vi "UHR-Fleezers Control (fpga) - Boltzmann 04-2018.vi"() -> ()   [LabVIEW 2013]
doc: "UHR-Fleezers Instrument Control Code (fpga)"
uses:
  <vilib>/eio/EIONode/EIONode.xnode
  <vilib>/eio/EIOMethodNode/EIOMethodNode.xnode
  <vilib>/rvi/DataTransferAndStorage/Container/XNode/niFpgaContainer.xnode
  <vilib>/Platform/TimedLoop/XDataNode/XDataNode.xnode
  <vilib>/Platform/TimedLoop/XDataNode/nitl_modes.ctl
  <vilib>/Platform/TimedLoop/XDataNode/XDNodeRunTimeDep.lvlib
  <vilib>/Platform/TimedLoop/XDataNode/wakeup.ctl
  <vilib>/Platform/TimedLoop/XDataNode/timing_clust.ctl
  <vilib>/addons/control/pid/fpga.llb/XNode/niFpgaPID.xnode
  <vilib>/rvi/eio/common/nirviEmuTemplateMethod_errors.vi
  <vilib>/rvi/interface/RandomDataEmulation/nirviRandomDataFpgaReadWriteTemplate.vi
panel:
  in  "Tab Control":T1(tab)=enum."Force FB"
  in  "Set 3":bool
  in  "Set 2":bool=TRUE
  in  "Set 1":bool=TRUE
  in  "Trap Pos to FIFO":bool
  in  "N of AI1 Int Acq Sets":i16=2 min=1 max=3 step=1
  out "AI Late Counter":u8
  in  "ai count":u16=400
  in  "+ phase":bool
  in  "Phase count adjustment":i16
  out "Relative phase":i16
  in  "AI to FIFO":bool
  out "BD1 Frequency Out 1":u64
  out "BD1 Frequency Out 2":u64
  out "Trap Pos FIFO Timeout":u16
  out "Trap AI FIFO Timeout":u16
  in  "Trap FIFO Set Timeout":i32
  in  "Tab Control 2":T2(tab)
  in  "Raster to target force":bool
  out "Actual Scan freq":u64
  out "BD1 measured amplitude 2":u16
  out "BD1 measured amplitude 1":u16
  in  "FB Offset":u16
  in  "FB Multi Factor":i16
  in  "Dynamic FB (Ronen)":bool
  in  "Negate Intensity FB":bool
  in  "RD":bool
  in  "FB1 output high":i16=3000
  in  "FB1 output low":i16
  in  "D1":i16
  in  "I1":i16=5
  in  "P1":i16=10
  in  "Swap F1 and F2":bool
  in  "Cont. Scan":bool
  in  "Abort scan":bool
  in  "Cycles per step":u64
  in  "Scan BD":bool
  in  "Number of scans":u16
  in  "Scan steps":u64
  in  "Scan freq.  increment":i64
  out "Scanning":bool
  in  "Start scan":bool
  in  "OSK Bd 1":bool
  in  "Reset Bd 1":bool
  in  "PMODE":bool
  in  "Direct RF Box \nCommunication":bool
  in  "Data BD 2":u8 format="%08b"
  in  "Data BD 1":u8 format="%08b"
  in  "Address":u8 format="%02x"
  in  "Update Data":bool
  in  "FPGA Controls\n RF Box":bool
  in  "Number Interlace Cycles":u8=2 min=1 max=3
  in  "Interlace Off Parameters":u8=1 min=1 max=3
  in  "Interlace ON/OFF":bool
  out "DIO Relative phase":i16
  in  "Phase count adjustment (DIO)":i16
  in  "+ phase (DIO)":bool
  out "DIO Late Counter":u8
  in  "DIO count 1 (ticks)":u16=400
  in  "DIO count 2 (ticks)":u16=400
  in  "DIO count 3 (ticks)":u16=400
  out "AI2 Y Sum Set 2":i16
  out "AI2 Y Sum Set 1":i16
  in  "FB Setpoint Set 1":i16 min=0 step=1
  in  "FB Reset Set 1":bool
  in  "FB On/Off Set 1":bool
  in  "FB Reset Set 2":bool
  in  "FB On/Off Set 2":bool
  in  "FB Setpoint Set 2":i16 min=0 step=1
  out "Scan I":u64
  in  "Amp switch delay":u8=5
  in  "Raster setpoint":fxp<+/-,16,1>
  in  "XY phase ext loop method":bool
  in  "BD 2 Amplitude 1":u16
  in  "BD 1 Amplitude 1":u16
  in  "BD 2 Frequency 1":u64
  in  "BD 1 Frequency 1":u64
  in  "BD 2 Amplitude 2":u16
  in  "BD 1 Amplitude 2":u16
  in  "BD 2 Frequency 2":u64
  in  "BD 1 Frequency 2":u64
  in  "BD 2 Amplitude 3":u16
  in  "BD 1 Amplitude 3":u16
  in  "BD 2 Frequency 3":u64
  in  "BD 1 Frequency 3":u64
  in  "BD 1 Delay (ticks)":u8
  in  "BD 2 Delay (Ticks)":u8 caption="Count(Ticks)"
  in  "Next trap write delay (ticks)":u8 caption="Count(Ticks)"
  in  "Trap 1 osc enable":bool
  in  "Trap 2 osc enable":bool
  in  "B factor":fxp<+/-,32,16>
  in  "FB Min frequency":u64
  in  "FB Max Frequency":u64
  in  "Dynamic Force FB (Ronen)":bool
  in  "FB2 output high":fxp<+/-,16,1>=0.999969482421875
  in  "FB2 output low":fxp<+/-,16,1>=-1.0
  in  "P2":fxp<+/-,16,8> format="%.11g"
  in  "I2":fxp<+/-,16,8>=10.0 format="%.11g"
  in  "D2":fxp<+/-,16,8> format="%.11g"
  in  "Negate Diff?":bool
  in  "Diff FB Measurement?":bool
  in  "FB Trig Integrate":u32=1
  out "TTrig?":bool
  in  "TTrig Negate Pos":bool=TRUE
  out "Trap Pos FB Int Signal":fxp<+/-,24,9> format="%.18g"
  out "Trap Pos FB Int-Norm Signal":fxp<+/-,16,1> format="%.16g"
  in  "FPGA TTrig Thresh":i64
  in  "FPGA Trap Trig":bool
  out "Trap Pos FB Action":i64
  in  "Trap Pos. FB Offset Factor":i64
  in  "Trap Pos. FB Mult Factor":i64=2
  in  "Trap Pos. FB Reset":bool
  in  "Trap Pos FB Monitor T1 or T2":bool
  in  "AI1 X Scale":u16
  in  "Trap Pos FB Int Count":u16=100
  in  "Trap Pos FB Negate Action":bool
  out "AI1 X Set 2":fxp<+/-,16,1>
  out "AI1 X Set 1":fxp<+/-,16,1>
  in  "Trap Pos. FB SP":fxp<+/-,16,1>
  in  "Force feedback":bool
  out "TTrig Sig":i64
  out "TTrig Fin Thresh":i64
  in  "1D or 2D Scan?":bool
  in  "Abort scan (MCL)":bool
  in  "MCL Scan Axis":bool
  in  "Cont. Scan (MCL)":bool
  out "Scan I (MCL)":u64
  in  "Number of scans (MCL)":u16
  out "Scanning MCL":bool
  in  "Scan steps (MCL)":u64
  in  "Cycles per step (MCL)":u64
  in  "Scan freq.  increment (MCL)":i16
  in  "Start scan (MCL)":bool
  in  "AO2":i16
  in  "AO1":i16
  out "MCL Late Counter":u8
  in  "MCL count":u32=800
  out "MCL Relative Phase":i16
  in  "Phase count adjustment (MCL)":i16
  in  "+ phase (MCL)":bool
  out "APD2 int gate":bool
  out "APD3 out state":bool
  in  "APD Gate Operating Mode":u8 max=2 step=1
  in  "Invert APD Gate":bool
  in  "APD Gate OFF Count":u16=100
  in  "APD Gate ON Count":u16=300
  out "APD 1 Gate Late Counter":u8
  out "APD 1 Gate Relative Phase":i16
  in  "Phase count adjustment (APD 1 Gate)":i16
  in  "+ phase (APD 1 Gate)":bool
  out "APD 2 Counts 0":u32
  out "APD 2 Counts 1":u32
  out "APD 1 Counts 0":u32
  out "APD 1 Counts 1":u32
  out "APD1 out state":bool
  in  "APD AO scale factor":i16=1
  in  "APD to FIFO":bool
  in  "APD Acq Rate Count":u32=20000000
  out "APD Acq Late Counter":u8
  out "APD Acq Relative Phase":i16
  in  "Phase Count Adjustment (APD Acq)":i16
  in  "+ phase (APD Acq)":bool
  in  "Phase count adjustment (APD 2 Gate)":i16
  out "APD 2 Gate Late Counter":u8
  out "APD 2 Gate Relative Phase":i16
  in  "+ phase (APD 2 Gate)":bool
  out "APD2 out state":bool
  out "APD 3 Counts 0":u32
  out "APD 3 Counts 1":u32
  out "APD 3 Gate Late Counter":u8
  in  "Phase count adjustment (APD 3 Gate)":i16
  out "APD 3 Gate Relative Phase":i16
  in  "+ phase (APD 3 Gate)":bool
  out "APD1 int gate":bool
  out "APD3 int gate":bool
  in  "D3":i16
  in  "I3":i16=5
  in  "P3":i16=10
  in  "Green Filter Flipper":bool
  in  "Green FB Count":u16=1200
  out "Green Late Counter":u8
  out "Green FB Relative Phase":i16
  in  "Phase count adjustment (Green FB)":i16=10
  in  "+ phase (Green FB)":bool
  out "Green FB Sum":i16
  in  "Green int current ON count adj":u16=150
  in  "Current Out":u16=30000
  in  "Green FB On/Off":bool
  in  "Green FB Setpoint":i16=250 min=0 step=1
  in  "Green FB Reset":bool
  in  "Operating Mode 2":u8=2 max=2 step=1
  in  "Invert GI 2":bool
  in  "Green interlace OFF count 2":u16=900
  in  "Green interlace ON count 2":u16=300
  out "GI Late Counter 2":u8
  out "GI Relative phase 2":i16
  in  "Phase count adjustment (GI) 2":i16=20
  in  "+ phase (GI) 2":bool
  in  "Green interlace OFF count":u16=100
  out "GI Relative phase":i16
  in  "Phase count adjustment (GI)":i16
  in  "+ phase (GI)":bool
  in  "Green interlace ON count":u16=300
  out "GI Late Counter":u8
  in  "Invert GI":bool
  in  "Operating Mode":u8 max=2 step=1
  in  "+ phase (RI)":bool
  out "RI Relative phase":i16
  out "RI Late Counter":u8
  in  "Red interlace ON count":u16=300
  in  "Red interlace OFF count":u16=100
  in  "Invert RI":bool
  in  "Red Laser Operating Mode":u8 max=2 step=1
  in  "Phase count adjustment (RI)":i16
  out "Red FB Intensity":i16
  in  "RI Current Out":u16=30000
  in  "Red FB On/Off":bool
  in  "D4":i16
  in  "I4":i16=5
  in  "P4":i16=10
  in  "Red FB Setpoint":i16=250 min=0 step=1
  in  "Red FB Reset":bool
  in  "RI Operating Mode 2":u8=2 max=2 step=1
  in  "Invert RI 2":bool
  in  "Phase count adjustment (BI AO)":i16=20
  in  "Blue current ON count adj (AO)":u16=150
  in  "BI Current Out":i16=30000
  in  "Blue FB On/Off":bool
  in  "D5":i16
  in  "I5":i16=5
  in  "P5":i16=10
  in  "Blue FB Setpoint":i16=250 min=0 step=1
  in  "Blue FB Reset":bool
  in  "BI Operating Mode (AO)":u8=2 max=2 step=1
  in  "Invert BI (AO)":bool
  in  "Blue OFF count (AO)":u16=900
  in  "Blue ON count (AO)":u16=300
  out "BI Late Counter (AO)":u8
  out "BI Relative phase (AO)":i16
  in  "+ phase (BI AO)":bool
  in  "Phase count adjustment (BI D)":i16
  in  "Blue Laser Operating Mode (D)":u8 max=2 step=1
  in  "Invert BI (D)":bool
  in  "Blue interlace OFF count (D)":u16=100
  in  "Blue interlace ON count (D)":u16=300
  out "Blue Late Counter (D)":u8
  out "BI Relative phase (D)":i16
  in  "+ phase (BI D)":bool
  out "Blue Intensity":i16
  # "Only one of these can be on\nat a time:"
  # "Raster Scan AOD"
  # "1 (X)"
  # "2 (Y)"
  # "IR Intensity Feedback (RF BD 1)"
  # "FB Gains Set 1"
  # "FB output range 1"
  # "False is usual, True is external loop method"
  # "Parameters if using the external RF switching loop"
  # "Parameters if using the usual internal RF switching method"
  # "FB Triggering Excitation Laser"
  # "Trap Pos. FB Gains"
  # "Trap Pos. FB Range"
  # "AO1 (Y)"
  # "2D"
  # "1D"
  # "AO2 (X)"
  # "APD AO for aligning"
  # "Detection Loop"
  # "Green fluorescent laser digital gate interlacing loop"
  # "0 Forced ON\n1 Forced OFF\n2 Interlacing"
  # "Green FB Gains"
  # "Red fluorescent laser digital gate interlacing loop"
  # "Detection Loop"
  # "0 Forced ON\n1 Forced OFF\n2 Interlacing"
  # "Analog/FB Control Loop\n(Disabled)"
  # "Digital Control Loop"
  # "Blue laser intensity reading"
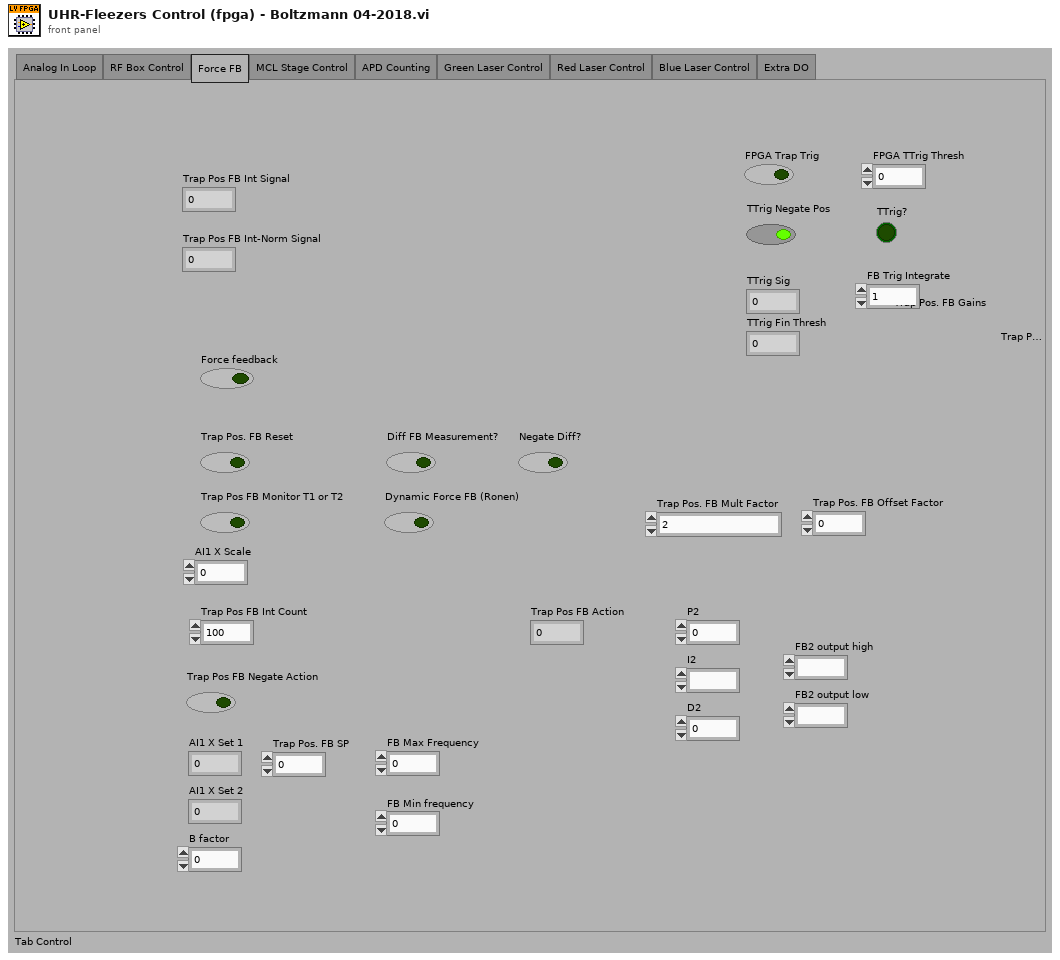
[diagram p1: front panel]
types:
  T1 = enum32{"Analog In Loop", "RF Box Control", "Force FB", "MCL Stage Control", "APD Counting", "Green Laser Control", "Red Laser Control", "Blue Laser Control", "Extra DO"}
  T2 = enum32{"Controls", "Interlacing Frequency and Amplitude Values", "Oscillate trap from memory"}
  T3 = typedef "XDNodeRunTimeDep.lvlib/timing_clust.ctl" = cluster{"Expected End [f-1]":u64, "Actual End [f-1]":u64, "Finished Late? [f-1]":bool, "Expected End [i-1]":u64, "Actual End [i-1]":u64, "Finished Late? [i-1]":bool, "Expected Start [i]":u64, "Actual Start [i]":u64, "Expected Start [f]":u64, "Actual Start [f]":u64, "Source Name":string, "Structure Name":string, "Period":i64, "Deadline":i64, "Offset":i64, "Start":i64, "Priority":i32, "Timeout":i32, "Mode":T4, "Wakeup Reason":T5, "Error":errorcluster, "Source Type":string, "Secondary Source Type":string, "Global End Time":u64, "Global Start Time":u64, "Frame Duration":u64, "Iteration Duration":u64, "Assigned CPU":i32, "I/O Scan Engine Mode":u32}
  T4 = typedef "XDNodeRunTimeDep.lvlib/nitl_modes.ctl" = enum32{"No Change", "Process missed periods, maintain original phase", "Discard missed periods, maintain original phase", "Process missed periods, ignore original phase", "Discard missed periods, ignore original phase"}
  T5 = typedef "XDNodeRunTimeDep.lvlib/wakeup.ctl" = enum32{"Normal", "Aborted", "Asynchronous wakeup", "Timing source error", "Timed loop error", "Timeout"}
  T6 = cluster{"proportional gain (Kc)":i16, "integral gain (Kc*Ts/Ti)":i16, "derivative gain (Kc*Td/Ts)":i16}
  T7 = cluster{"FB1 output high":i16, "FB1 output low":i16}
  T8 = cluster{"P2":fxp<+/-,16,8>, "I2":fxp<+/-,16,8>, "D2":fxp<+/-,16,8>}
  T9 = cluster{"FB2 output high":fxp<+/-,16,1>, "FB2 output low":fxp<+/-,16,1>}
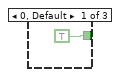
[diagram p2: hidden frame]
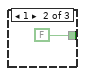
[diagram p3: hidden frame]
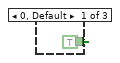
[diagram p4: hidden frame]
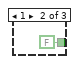
[diagram p5: hidden frame]
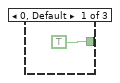
[diagram p7: hidden frame]
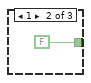
[diagram p8: hidden frame]
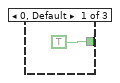
[diagram p10: hidden frame]
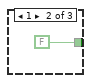
[diagram p11: hidden frame]
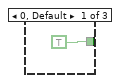
[diagram p14: hidden frame]
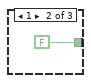
[diagram p15: hidden frame]
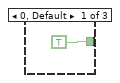
[diagram p17: hidden frame]
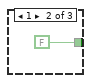
[diagram p18: hidden frame]
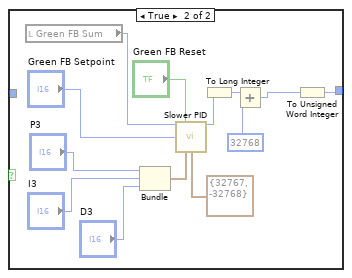
[diagram p20: hidden frame]
diagram:
  w7 = FALSE
  w5 = FALSE
  # "timing array current index"
  # "timing array"
  # "timing counter (phase adjusted here)"
  # "late counter"
  n1 = flat-sequence "FPGA initialization to do before running any of the loops" {
    tunnel: [u16 0 ("DIO count 3 (ticks)")] -> w4
    tunnel: [w15] -> _
    frame #0 {
      w14 = FALSE ("Enable")
      # "BD 2 (Y)"
      # "BD 1 (X)"
      # "Start up expansion chassis early\nto avoid delays later"
      # "This pin controls udclk on the RF boards.\nWhen initially configuring the boards, this pin needs to be\nconfigured as a high impedance input.  Later it will be switched\nto an output."
      # "Initial setting of DIO data and \naddress to low (before reset).  \nThis needs to happen before the other\ncontrol method loops execute."
      n2 = xnode "FPGA I/O Node"("Chassis2/Mod1/AO0"=u16 0 ("Chassis2/Mod4/AO0")) -> ("Chassis2/Mod2/AI0"=w15:i16)  [unwired: 2 in, 2 out]
      n3 = xnode "FPGA I/O Method Node"("Enable"=w14) -> ()  [unwired: 1 in, 1 out]
      n4 = xnode "FPGA I/O Method Node"("Enable"=w14) -> ()  [unwired: 1 in, 1 out]
      n5 = xnode "FPGA I/O Node"("Connector1/DIO0"=FALSE, "Connector1/DIO1"=FALSE, "Connector1/DIO2"=FALSE, "Connector1/DIO3"=FALSE, "Connector1/DIO4"=FALSE, "Connector1/DIO5"=FALSE, "Connector1/DIO6"=FALSE, "Connector1/DIO7"=FALSE, "Connector1/DIO8"=FALSE, "Connector1/DIO9"=FALSE, "Connector1/DIO10"=FALSE, "Connector1/DIO11"=FALSE, "Connector1/DIO12"=FALSE, "Connector1/DIO13"=FALSE, "Connector1/DIO15"=FALSE, "Connector1/DIO20"=FALSE, "Connector1/DIO21"=FALSE, "Connector1/DIO22"=FALSE, "Connector1/DIO23"=FALSE, "Connector1/DIO24"=FALSE, "Connector1/DIO25"=FALSE, "Connector1/DIO26"=FALSE, "Connector1/DIO27"=FALSE, "Connector1/DIO14"=FALSE) -> ()  [unwired: 24 in, 24 out]
    }
  }
  n6 = local read "AO1"() -> (w12:i16)
  n7 = local read "AO2"() -> (w11:i16)
  n8 = node-c288() -> (w10:T3)  [unwired: 1 in]
  n9 = To Unsigned Long Integer(number=w4) -> (unsigned 32bit integer=w8:u32)
  n10 = timed-loop "RF box board DIO control: control bits" {
    timing: w10 -> [_]
    timing-out: [_] -> w9
    tunnel: [w44] -> _
    tunnel: w4 -> [w44]
    stop <- FALSE stop-if-true
    n11 = xnode "FPGA I/O Node"("Connector1/DIO16"="RD", "Connector1/DIO17"="PMODE", "Connector1/DIO18"="OSK Bd 1", "Connector1/DIO19"="Reset Bd 1", "Connector0/DIO3"="Green Filter Flipper") -> ()  [unwired: 5 in, 5 out]
  }
  n12 = disable-structure shown="Disabled" {
    disable-tunnel: w7 -> [w52 _]
    disable-tunnel: w4 -> [w51 _]
    frame Disabled {
      n13 = while "APD 2 Gating" {
        shift-right: [w56] -> _
        shift-left: w51 -> [w61]
        shift-right: [w55] -> _
        shift-left: w52 -> [w53]
        stop <- FALSE stop-if-true
        n14 = flat-sequence {
          tunnel: w61 -> [w64]
          tunnel: [w65] -> w59
          tunnel: [w64] -> w57
          tunnel: [w63] -> w54
          tunnel: w53 -> [w63]
          tunnel: [w68] -> w60
          tunnel: w59 -> [w68]
          tunnel: [w67] -> w58
          tunnel: w57 -> [w67]
          tunnel: w54 -> [w66]
          tunnel: [w90] -> w56
          tunnel: w60 -> [w100]
          tunnel: w58 -> [w98]
          tunnel: [w69] -> w55
          frame #0 {
            n15 = call "Loop Timer8"("Count(Ticks)"=w64) -> ("Tick Count(Ticks)"=w65:u16)
          }
          frame #1 {
            # "Signal maybe then sent through \na transistor before APD"
            n16 = xnode "FPGA I/O Node"("Connector0/DIO8"=w66, "Connector0/DIO9"=w66, "Connector0/DIO10"=w66, "Connector0/DIO11"=w66) -> ()  [unwired: 4 in, 4 out]
            "APD2 int gate" <- w66
          }
          frame #2 {
            n17 = local read "APD Gate ON Count"() -> (w83:u16)
            n18 = local read "APD Gate OFF Count"() -> (w82:u16)
            n19 = feedback #1(TRUE) -> (w95:bool)
            n20 = feedback-in #2(w100) -> ()
            n21 = feedback #2(w100) -> (w84:u16)
            n22 = Not(x=w95) -> (.not. x?=w93:bool)
            n23 = feedback-in #1(w93) -> ()
            n24 = Subtract(x=w100, y=w84) -> (x-y=w99:u16)
            n25 = Select(t=w83, s=w93, f=w82) -> (s? t:f=w97:u16)
            n26 = Subtract(x=w99, y=w98) -> (x-y=w75:u16)
            n27 = Subtract(x=w97, y=w75) -> (x-y=w89:u16)
            n28 = Number To Boolean Array(number=w75) -> (Boolean array=w74:bool[])
            n29 = Or Array Elements(Boolean array=w74) -> (logical OR=w73:bool)
            n30 = Boolean To (0,1)(Boolean="+ phase (APD 2 Gate)") -> (0, 1=w87:i16)
            n31 = Multiply(x=w87, y="Phase count adjustment (APD 2 Gate)") -> (x*y=w85:i16)
            n32 = Boolean To (0,1)(Boolean=w73) -> (0, 1=w80:i16)
            n33 = Add(x=w89, y=w85) -> (x+y=w90:u16)
            n34 = To Unsigned Byte Integer(number=w80) -> (unsigned 8bit integer=w77:u8)
            n35 = feedback #3(i16 0) -> (w92:i16)
            n36 = Subtract(x=w92, y=w85) -> (x-y=w91:i16)
            "APD 2 Gate Relative Phase" <- w91
            n37 = feedback-in #3(w91) -> ()
            n38 = feedback #4(u8 0) -> (w78:u8)
            n39 = Add(x=w77, y=w78) -> (x+y=w76:u8)
            "APD 2 Gate Late Counter" <- w76
            n40 = feedback-in #4(w76) -> ()
            n41 = local read "APD Gate Operating Mode"() -> (w81:u8)
            n42 = case shown="2" w81 {
              tunnel: [TRUE FALSE w103] -> w70
              tunnel: w95 -> [_ _ w103]
              frame 0, Default {
              }
              frame 1 {
              }
              frame 2 {
              }
            }
            n43 = local read "Invert APD Gate"() -> (w72:bool)
            n44 = Not(x=w70) -> (.not. x?=w71:bool)
            n45 = Select(t=w71, s=w72, f=w70) -> (s? t:f=w69:bool)
          }
        }
      }
      n46 = while "APD 1 Gating" {
        shift-right: [w107] -> _
        shift-left: w51 -> [w112]
        shift-right: [w106] -> _
        shift-left: w52 -> [w104]
        stop <- FALSE stop-if-true
        n47 = flat-sequence {
          tunnel: w112 -> [w115]
          tunnel: [w116] -> w110
          tunnel: [w115] -> w108
          tunnel: [w114] -> w105
          tunnel: w104 -> [w114]
          tunnel: [w119] -> w111
          tunnel: w110 -> [w119]
          tunnel: [w118] -> w109
          tunnel: w108 -> [w118]
          tunnel: w105 -> [w117]
          tunnel: [w137] -> w107
          tunnel: w111 -> [w151]
          tunnel: w109 -> [w148]
          tunnel: [w120] -> w106
          frame #0 {
            n48 = call "Loop Timer7"("Count(Ticks)"=w115) -> ("Tick Count(Ticks)"=w116:u16)
          }
          frame #1 {
            # "Signal maybe then sent through \na transistor before APD"
            n49 = xnode "FPGA I/O Node"("Connector0/DIO4"=w117, "Connector0/DIO5"=w117, "Connector0/DIO6"=w117, "Connector0/DIO7"=w117) -> ()  [unwired: 4 in, 4 out]
            "APD1 int gate" <- w117
          }
          frame #2 {
            n50 = feedback #5(TRUE) -> (w143:bool)
            n51 = feedback-in #6(w151) -> ()
            n52 = feedback #6(w151) -> (w150:u16)
            n53 = Not(x=w143) -> (.not. x?=w140:bool)
            n54 = feedback-in #5(w140) -> ()
            n55 = Subtract(x=w151, y=w150) -> (x-y=w149:u16)
            n56 = Select(t="APD Gate ON Count", s=w140, f="APD Gate OFF Count") -> (s? t:f=w145:u16)
            n57 = Subtract(x=w149, y=w148) -> (x-y=w125:u16)
            n58 = Subtract(x=w145, y=w125) -> (x-y=w136:u16)
            n59 = Number To Boolean Array(number=w125) -> (Boolean array=w126:bool[])
            n60 = Or Array Elements(Boolean array=w126) -> (logical OR=w124:bool)
            n61 = Boolean To (0,1)(Boolean="+ phase (APD 1 Gate)") -> (0, 1=w134:i16)
            n62 = Boolean To (0,1)(Boolean=w124) -> (0, 1=w131:i16)
            n63 = Multiply(x=w134, y="Phase count adjustment (APD 1 Gate)") -> (x*y=w132:i16)
            n64 = To Unsigned Byte Integer(number=w131) -> (unsigned 8bit integer=w128:u8)
            n65 = Add(x=w136, y=w132) -> (x+y=w137:u16)
            n66 = feedback #7(i16 0) -> (w139:i16)
            n67 = Subtract(x=w139, y=w132) -> (x-y=w138:i16)
            "APD 1 Gate Relative Phase" <- w138
            n68 = feedback-in #7(w138) -> ()
            n69 = feedback #8(u8 0) -> (w129:u8)
            n70 = Add(x=w128, y=w129) -> (x+y=w127:u8)
            "APD 1 Gate Late Counter" <- w127
            n71 = feedback-in #8(w127) -> ()
            n72 = case shown="2" "APD Gate Operating Mode" {
              tunnel: [TRUE FALSE w154] -> w121
              tunnel: w143 -> [_ _ w154]
              frame 0, Default {
              }
              frame 1 {
              }
              frame 2 {
              }
            }
            n73 = Not(x=w121) -> (.not. x?=w122:bool)
            n74 = Select(t=w122, s="Invert APD Gate", f=w121) -> (s? t:f=w120:bool)
          }
        }
      }
    }
    frame Enabled {
    }
  }
  n75 = while "RF box board direct communication loop" {
    tunnel: w4 -> [_]
    stop <- FALSE stop-if-true
    n76 = case "Whether to use direct communication method (only use one method at a time)" shown="True" "Direct RF Box \nCommunication" {
      frame False {
      }
      frame True {
        n77 = case shown="True" "Update Data" {
          frame False {
          }
          frame True {
            n78 = flat-sequence {
              frame #0 {
                n79 = First Call?() -> (First Call?: T/F=w158:bool)
                n80 = case shown="True" w158 {
                  frame False {
                  }
                  frame True {
                    # "If first time data updated, be sure to set WR high\nbefore setting data and address bits."
                    n81 = flat-sequence {
                      frame #0 {
                        n82 = xnode "FPGA I/O Node"("Connector1/DIO15"=TRUE) -> ()  [unwired: 1 in, 1 out]
                      }
                      frame #1 {
                        n83 = call "Wait"("Count(Ticks)"=u8 40 ("DO Delay 3 (Ticks)")) -> ()  [unwired: 1 out]
                      }
                    }
                  }
                }
              }
              frame #1 {
                n84 = Number To Boolean Array(number="Address") -> (Boolean array=w207:bool[])
                n85 = Number To Boolean Array(number="Data BD 1") -> (Boolean array=w208:bool[])
                n86 = Number To Boolean Array(number="Data BD 2") -> (Boolean array=w177:bool[])
                n87 = Index Array(array=w208, index=7) -> (element=w192:bool)
                n88 = Index Array(array=w208, index=6) -> (element=w191:bool)
                n89 = Index Array(array=w208, index=5) -> (element=w190:bool)
                n90 = Index Array(array=w208, index=4) -> (element=w189:bool)
                n91 = Index Array(array=w208, index=3) -> (element=w188:bool)
                n92 = Index Array(array=w208, index=2) -> (element=w187:bool)
                n93 = Index Array(array=w208, index=1) -> (element=w186:bool)
                n94 = Index Array(array=w208, index=0) -> (element=w185:bool)
                n95 = Index Array(array=w207, index=5) -> (element=w184:bool)
                n96 = Index Array(array=w207, index=4) -> (element=w183:bool)
                n97 = Index Array(array=w207, index=3) -> (element=w182:bool)
                n98 = Index Array(array=w207, index=2) -> (element=w181:bool)
                n99 = Index Array(array=w207, index=1) -> (element=w180:bool)
                n100 = Index Array(array=w207, index=0) -> (element=w179:bool)
                n101 = Index Array(array=w177, index=7) -> (element=w168:bool)
                n102 = Index Array(array=w177, index=6) -> (element=w167:bool)
                n103 = Index Array(array=w177, index=5) -> (element=w166:bool)
                n104 = Index Array(array=w177, index=4) -> (element=w165:bool)
                n105 = Index Array(array=w177, index=3) -> (element=w164:bool)
                n106 = Index Array(array=w177, index=2) -> (element=w163:bool)
                n107 = Index Array(array=w177, index=1) -> (element=w162:bool)
                n108 = Index Array(array=w177, index=0) -> (element=w161:bool)
                n109 = xnode "FPGA I/O Node"("Connector1/DIO0"=w192, "Connector1/DIO1"=w191, "Connector1/DIO2"=w190, "Connector1/DIO3"=w189, "Connector1/DIO4"=w188, "Connector1/DIO5"=w187, "Connector1/DIO6"=w186, "Connector1/DIO7"=w185, "Connector1/DIO8"=w184, "Connector1/DIO9"=w183, "Connector1/DIO10"=w182, "Connector1/DIO11"=w181, "Connector1/DIO12"=w180, "Connector1/DIO13"=w179, "Connector1/DIO20"=w168, "Connector1/DIO21"=w167, "Connector1/DIO22"=w166, "Connector1/DIO23"=w165, "Connector1/DIO24"=w164, "Connector1/DIO25"=w163, "Connector1/DIO26"=w162, "Connector1/DIO27"=w161) -> ()  [unwired: 22 in, 22 out]
              }
              frame #2 {
                # "wait and then apply write signal"
                n110 = call "Wait2"("Count(Ticks)"=u8 40 ("DO Delay 1 (Ticks)")) -> ()  [unwired: 1 out]
              }
              frame #3 {
                # "sending bit low writes data to board buffer"
                n111 = xnode "FPGA I/O Node"("Connector1/DIO15"=FALSE) -> ()  [unwired: 1 in, 1 out]
              }
              frame #4 {
                # "wait then return write signal"
                n112 = call "Wait3"("Count(Ticks)"=u8 40 ("DO Delay 2 (Ticks)")) -> ()  [unwired: 1 out]
              }
              frame #5 {
                # "sending bit high makes ready to\nwrite more data"
                n113 = xnode "FPGA I/O Node"("Connector1/DIO15"=TRUE) -> ()  [unwired: 1 in, 1 out]
              }
            }
          }
        }
      }
    }
  }
  n114 = while "RF box board DIO control: parallel communication" {
    shift-right: [w227] -> _
    shift-left: w4 -> [w226]
    shift-right: [w225] -> _
    shift-left: FALSE ("Swap F1 and F2") -> [w224]
    shift-right: [w219] -> _
    shift-left: u16 0 -> [w220]
    shift-right: [w217] -> _
    shift-left: u16 0 -> [w218]
    shift-right: [w215] -> _
    shift-left: u64 0 -> [w216]
    stop <- FALSE stop-if-true
    n115 = flat-sequence {
      tunnel: w224 -> [w231]
      tunnel: w226 -> [w229]
      tunnel: [w231] -> w223
      tunnel: [w230] -> w222
      tunnel: [w229] -> w221
      tunnel: [w243] -> w227
      tunnel: [w242] -> w225
      tunnel: w223 -> [w241]
      tunnel: w222 -> [w239]
      tunnel: w221 -> [w238]
      tunnel: w220 -> [w237]
      tunnel: [w236] -> w219
      tunnel: w218 -> [w235]
      tunnel: [w234] -> w217
      tunnel: w216 -> [w233]
      tunnel: [w232] -> w215
      frame #0 {
        n116 = call "Loop Timer"("Count(Ticks)"=w229) -> ("Tick Count(Ticks)"=w230:u16)
      }
      frame #1 {
        n117 = flat-sequence {
          tunnel: ["FPGA Controls\n RF Box"] -> w240
          tunnel: w241 -> [w244]
          tunnel: [w307] -> w243
          tunnel: [w320] -> w242
          tunnel: w240 -> [w319]
          tunnel: w239 -> [w313]
          tunnel: w238 -> [w310]
          tunnel: w237 -> [w276]
          tunnel: [w275] -> w236
          tunnel: w235 -> [w272]
          tunnel: [w271] -> w234
          tunnel: w233 -> [w270]
          tunnel: [w269] -> w232
          frame #0 {
            n118 = case shown="True" "FPGA Controls\n RF Box" {
              tunnel: w244 -> [_ w246]
              frame False {
              }
              frame True {
                n119 = flat-sequence {
                  tunnel: w246 -> [w256]
                  frame #0 {
                    n120 = First Call?() -> (First Call?: T/F=w247:bool)
                    n121 = case shown="True" w247 {
                      frame False {
                      }
                      frame True {
                        # "BD 2"
                        # "BD 1"
                        # "If first time data updated, be sure to set WR high and UDCLK low\nbefore setting data and address bits."
                        n122 = xnode "FPGA I/O Method Node"("Enable"=TRUE) -> ("FPGA I/O Out"=w249:refnum<k21>)  [unwired: 1 in]
                        n123 = xnode "FPGA I/O Method Node"("Enable"=TRUE) -> ("FPGA I/O Out"=w252:refnum<k21>)  [unwired: 1 in]
                        n124 = xnode "FPGA I/O Node"("Connector1/DIO15"=TRUE) -> ()  [unwired: 1 in, 1 out]
                        n125 = xnode "FPGA I/O Node"("I/O Item"=FALSE ("Connector1/DIO30"), "FPGA I/O In"=w249) -> ()  [unwired: 1 out]
                        n126 = xnode "FPGA I/O Node"("I/O Item"=FALSE ("Connector1/DIO30"), "FPGA I/O In"=w252) -> ()  [unwired: 1 out]
                      }
                    }
                  }
                  frame #1 {
                    n127 = case shown="False" FALSE {
                      tunnel: w256 -> [w258 _]
                      frame False {
                        # "Usual operation"
                        n128 = flat-sequence "BD 1 (X)" {
                          tunnel: w258 -> [w265]
                          tunnel: "Amp switch delay" -> [w266]
                          frame #0 {
                            n129 = call "Wait6"("Count(Ticks)"="BD 1 Delay (ticks)") -> ()  [unwired: 1 out]
                          }
                          frame #1 {
                            # "switch frequency"
                            n130 = xnode "FPGA I/O Node"("Connector1/DIO36"=w265) -> ()  [unwired: 1 in, 1 out]
                          }
                          frame #2 {
                            # "~5 ticks is usual"
                            n131 = call "Wait4"("Count(Ticks)"=w266) -> ()  [unwired: 1 out]
                          }
                          frame #3 {
                            # "this switches amplitude"
                            # "switch amplitude"
                            # "send udclk high"
                            n132 = xnode "FPGA I/O Node"("Connector1/DIO30"=TRUE ("Connector1/DIO15")) -> ()  [unwired: 1 in, 1 out]
                          }
                          frame #4 {
                            # "reset to be ready for next\ncycle"
                            # "send udclk low"
                            n133 = xnode "FPGA I/O Node"("Connector1/DIO30"=FALSE ("Connector1/DIO15")) -> ()  [unwired: 1 in, 1 out]
                          }
                        }
                        n134 = flat-sequence "BD 2 (Y)" {
                          tunnel: w258 -> [w260]
                          tunnel: "Amp switch delay" -> [w261]
                          frame #0 {
                            n135 = call "Wait7"("Count(Ticks)"="BD 2 Delay (Ticks)") -> ()  [unwired: 1 out]
                          }
                          frame #1 {
                            # "switch frequency"
                            n136 = xnode "FPGA I/O Node"("Connector1/DIO37"=w260) -> ()  [unwired: 1 in, 1 out]
                          }
                          frame #2 {
                            # "~5 ticks is usual"
                            n137 = call "PID (FPGA).vi3"("Count(Ticks)"=w261) -> ()  [unwired: 1 out]
                          }
                          frame #3 {
                            # "this switches amplitude"
                            # "switch amplitude"
                            # "send udclk high"
                            n138 = xnode "FPGA I/O Node"("Connector1/DIO29"=TRUE ("Connector1/DIO15")) -> ()  [unwired: 1 in, 1 out]
                          }
                          frame #4 {
                            # "reset to be ready for next\ncycle"
                            # "send udclk low"
                            n139 = xnode "FPGA I/O Node"("Connector1/DIO29"=FALSE ("Connector1/DIO15")) -> ()  [unwired: 1 in, 1 out]
                          }
                        }
                      }
                      frame True {
                        # "Operation when you need a long delay for either X or Y to synchonize AOD light out phase (> ~100 ticks)."
                        # "Trigger the external loop by sending the boolean FSK value through a FIFO"
                      }
                    }
                  }
                }
              }
            }
          }
          frame #1 {
            # "This is the prior cycle's on time"
            # "increment timing\nindex, reset to 0 if \nend of matrix"
            # "Reset to begginning (1) when number of cycles reached."
            # "timing index"
            # "build byte stacks for writing data\n(must correspond to addresses array constant)"
            # "Timing housekeeping"
            # "Adjust phase if late\n(maintains constant phase relationship between cycles)"
            n140 = Bundle("FB1 output high"="FB1 output high", "FB1 output low"="FB1 output low") -> (w280:T7)  [unwired: 1 in]
            n141 = Bundle("P1"="P1", "I1"="I1", "D1"="D1") -> (w281:cluster{"P1":i16, "I1":i16, "D1":i16})  [unwired: 1 in]
            n142 = feedback #9(u8 0 ("t")) -> (w316:u8)
            n143 = Increment(x=w316) -> (x+1=w359:u8)
            n144 = Increment(x="Number Interlace Cycles") -> (x+1=w354:u8)
            n145 = Equal?(x=w359, y=w354) -> (x = y?=w361:bool)
            n146 = Select(t=u8 1, s=w361, f=w359) -> (s? t:f=w315:u8)
            n147 = feedback-in #9(w315) -> ()
            n148 = Increment(x=w315) -> (x+1=w356:u8)
            n149 = Equal?(x=w356, y=w354) -> (x = y?=w357:bool)
            n150 = Select(t=u8 1, s=w357, f=w356) -> (s? t:f=w353:u8)
            n151 = Select(t=w353, s="Interlace ON/OFF", f="Interlace Off Parameters") -> (s? t:f=w279:u8)
            n152 = case shown="1, Default" w279 {
              tunnel: [w409 w689 "BD 1 Frequency 3"] -> w349
              tunnel: [w453 "BD 2 Frequency 2" "BD 2 Frequency 3"] -> w338
              tunnel: ["BD 2 Amplitude 1" "BD 2 Amplitude 2" "BD 2 Amplitude 3"] -> w295
              tunnel: [w408 w680 "BD 1 Amplitude 3"] -> w298
              tunnel: w281 -> [w428 w691 _]
              tunnel: w280 -> [w429 w690 _]
              tunnel: "Negate Intensity FB" -> [w427 w687 _]
              tunnel: "Dynamic FB (Ronen)" -> [w426 w686 _]
              tunnel: w276 -> [w423 w685 w737]
              tunnel: [w408 w685 w737] -> w275
              tunnel: "FB Multi Factor" -> [w422 w683 _]
              tunnel: "FB Offset" -> [w421 w682 _]
              tunnel: w272 -> [w420 w684 w736]
              tunnel: [w420 w680 w736] -> w271
              tunnel: w270 -> [w407 w681 w735]
              tunnel: [w409 w681 w735] -> w269
              frame 1, Default {
                w441 = fxp<+/-,24,9> 0.0 ("AI1 X Set 2")
                w436 = u16 0
                w449 = u64 0 ("f")
                # "Changed by Ronen - Added\nB factor to weight in ratio between\nAlphas and Kappa for truly correct\ndetermination of average force"
                # "Added by Ronen -\nUpper and Lower \nLimits for the FB \ngenerated frequency\nto avoid losing bead \nwhen tether breaks"
                # "Changed by Ronen - correction \nby PID is now implemented not on \nthe Base BD1 frequency but on the last\nfrequency sent."
                # "BD1 Amp 1"
                # "Changed by Ronen-\n FB changed \nso that value from PID is added to\nlast amplitude sent to board. Correction\nValue can be scaled down same as the force\nFB value."
                # "This signal integration happens no matter what\nso that correct setpoints can be chosen before \nturning on the FB."
                # "Trap 1"
                n153 = local read "AI1 X Set 2"() -> (w415:fxp<+/-,16,1>)
                n154 = local read "Scanning"() -> (w454:bool)
                n155 = local read "AI1 X Set 1"() -> (w439:fxp<+/-,16,1>)
                n156 = Multiply(x=w415, y="B factor") -> (x*y=w413:fxp<+/-,48,17>)
                n157 = Or(x=w454, y="Start scan") -> (x .or. y?=w406:bool)
                n158 = case shown="True" "Diff FB Measurement?" {
                  tunnel: w413 -> [w475 w484]
                  tunnel: w439 -> [w474 w485]
                  tunnel: [w472 w476] -> w401
                  frame False {
                    n159 = Select(t=w474, s="Trap Pos FB Monitor T1 or T2", f=w475) -> (s? t:f=w472:fxp<+/-,48,17>)
                  }
                  frame True {
                    n160 = Subtract(x=w485, y=w484) -> (x-y=w477:fxp<+/-,48,17>)
                    n161 = Not(x="Negate Diff?") -> (.not. x?=w483:bool)
                    n162 = Boolean To (0,1)(Boolean="Negate Diff?") -> (0, 1=w481:i16)
                    n163 = Boolean To (0,1)(Boolean=w483) -> (0, 1=w482:i16)
                    n164 = Negate(x=w481) -> (-x=w480:i16)
                    n165 = Add(x=w480, y=w482) -> (x+y=w478:i16)
                    n166 = Multiply(x=w478, y=w477) -> (x*y=w476:fxp<+/-,63,32>)
                  }
                }
                n167 = feedback #10(w436) -> (w435:u16)
                n168 = Increment(x=w435) -> (x+1=w437:u16)
                n169 = Greater Or Equal?(x=w437, y="Trap Pos FB Int Count") -> (x >= y?=w419:bool)
                n170 = Select(t=w436, s=w419, f=w437) -> (s? t:f=w438:u16)
                n171 = feedback-in #10(w438) -> ()
                n172 = feedback #11(w441) -> (w440:fxp<+/-,24,9>)
                n173 = Add(x=w401, y=w440) -> (x+y=w434:fxp<+/-,24,9>)
                n174 = Select(t=w441, s=w419, f=w434) -> (s? t:f=w444:fxp<+/-,24,9>)
                n175 = feedback-in #11(w444) -> ()
                n176 = case "For intensity feedback" shown="True" "FB On/Off Set 1" {
                  tunnel: w423 -> [_ w644]
                  tunnel: ["BD 1 Amplitude 1" w650] -> w408
                  tunnel: w429 -> [_ w651]
                  tunnel: w428 -> [_ w652]
                  tunnel: w427 -> [_ w649]
                  tunnel: w426 -> [_ w648]
                  tunnel: w422 -> [_ w643]
                  tunnel: w421 -> [_ w642]
                  frame False {
                  }
                  frame True {
                    n177 = local read "AI2 Y Sum Set 1"() -> (w646:i16)
                    n178 = case shown="True" w648 {
                      tunnel: w652 -> [w658 w672]
                      tunnel: w651 -> [w659 w671]
                      tunnel: [w653 w670] -> w650
                      tunnel: w649 -> [_ w669]
                      tunnel: "FB Setpoint Set 1" -> [w657 w668]
                      tunnel: w646 -> [w656 w667]
                      tunnel: "FB Reset Set 1" -> [w655 w666]
                      tunnel: w644 -> [_ w665]
                      tunnel: w643 -> [_ w663]
                      tunnel: w642 -> [_ w661]
                      frame False {
                        n179 = call "Slower PID.vi"("process variable"=w656, "reset?"=w655, "setpoint"=w657, "PID gains (x 2^8)"=w658, "output range"=w659) -> ("output"=w654:i16)  [unwired: 10 out]
                        n180 = To Unsigned Word Integer(number=w654) -> (unsigned 16bit integer=w653:u16)
                      }
                      frame True {
                        n181 = call "Slower PID.vi"("process variable"=w667, "reset?"=w666, "setpoint"=w668, "PID gains (x 2^8)"=w672, "output range"=w671) -> ("output"=w673:i16)  [unwired: 10 out]
                        n182 = To Unsigned Word Integer(number=w673) -> (unsigned 16bit integer=w664:u16)
                        n183 = Scale By Power Of 2(n=w663, x=w664) -> (x*2^n=w662:u16)
                        n184 = Add(x=w662, y=w661) -> (x+y=w660:u16)
                        n185 = case shown="True" w669 {
                          tunnel: w660 -> [w676 w678]
                          tunnel: w665 -> [w674 w679]
                          tunnel: [w675 w677] -> w670
                          frame False {
                            n186 = Add(x=w674, y=w676) -> (x+y=w675:u16)
                          }
                          frame True {
                            n187 = Subtract(x=w679, y=w678) -> (x-y=w677:u16)
                          }
                        }
                      }
                    }
                  }
                }
                "BD1 measured amplitude 1" <- w408
                n188 = Divide(x=w434, y="Trap Pos FB Int Count") -> (x/y=w400:fxp<+/-,16,1>)
                n189 = case "For raster scanning" shown="True" w406 {
                  tunnel: [u64 0 w595] -> w450
                  tunnel: "Start scan" -> [_ w590]
                  tunnel: [FALSE w582] -> w405
                  tunnel: [i16 0 w581] -> w402
                  tunnel: w400 -> [_ w580]
                  frame False {
                    n190 = local write "Scanning"(FALSE ("scanning")) -> ()
                  }
                  frame True {
                    w588 = u64 0
                    # "Changed by RG, to introduce force\ndependent stopping of the raster scan \nand manual stopping"
                    # "count number of cycles"
                    n191 = feedback #12(w588) -> (w592:u64)
                    n192 = Select(t=w588, s=w590, f=w592) -> (s? t:f=w594:u64)
                    n193 = Increment(x=w594) -> (x+1=w586:u64)
                    n194 = Equal?(x=i16 1, y=w586) -> (x = y?=w584:bool)
                    n195 = And(x="Abort scan", y=w584) -> (x .and. y?=w582:bool)
                    n196 = Greater?(x="Cycles per step", y=w586) -> (0:w589:bool)
                    n197 = Select(t=w586, s=w589, f=w588) -> (s? t:f=w591:u64)
                    n198 = feedback-in #12(w591) -> ()
                    n199 = Greater?(x=w580, y="Raster setpoint") -> (0:w577:bool)
                    n200 = And(x=w577, y="Raster to target force") -> (x .and. y?=w575:bool)
                    n201 = case shown="False" w582 {
                      tunnel: [w602 i16 0] -> w595
                      tunnel: w590 -> [w627 _]
                      tunnel: w589 -> [w620 _]
                      tunnel: w588 -> [w610 _]
                      tunnel: [w604 FALSE] -> w583
                      tunnel: [w600 w638] -> w581
                      tunnel: [w603 w639] -> w578
                      frame False {
                        w611 = i64 0
                        # "scan incr."
                        # "freq. incr. mult."
                        # "count steps"
                        n202 = feedback #13(w610) -> (w635:u64)
                        n203 = Select(t=w610, s=w627, f=w635) -> (s? t:f=w603:u64)
                        n204 = Increment(x=w603) -> (x+1=w634:u64)
                        n205 = Add(x="Scan steps", y="Scan steps") -> (x+y=w633:u64)
                        n206 = Select(t=w603, s=w620, f=w634) -> (s? t:f=w615:u64)
                        n207 = Greater?(x=w633, y=w615) -> (0:w614:bool)
                        n208 = Select(t=w615, s=w614, f=w610) -> (s? t:f=w631:u64)
                        n209 = feedback-in #13(w631) -> ()
                        n210 = Equal?(x="Scan steps", y=w615) -> (x = y?=w619:bool)
                        n211 = Greater?(x="Scan steps", y=w603) -> (0:w630:bool)
                        n212 = feedback #14(w611) -> (w632:i64)
                        n213 = Select(t=w611, s=w627, f=w632) -> (s? t:f=w617:i64)
                        n214 = Increment(x=w617) -> (x+1=w629:i64)
                        n215 = Decrement(x=w617) -> (x-1=w628:i64)
                        n216 = Select(t=w629, s=w630, f=w628) -> (s? t:f=w618:i64)
                        n217 = Select(t=w617, s=w619, f=w618) -> (s? t:f=w616:i64)
                        n218 = Select(t=w617, s=w620, f=w616) -> (s? t:f=w612:i64)
                        n219 = Select(t=w612, s=w614, f=w611) -> (s? t:f=w613:i64)
                        n220 = feedback-in #14(w613) -> ()
                        n221 = feedback #15(w610) -> (w626:u64)
                        n222 = Select(t=w610, s=w627, f=w626) -> (s? t:f=w622:u64)
                        n223 = Increment(x=w622) -> (x+1=w623:u64)
                        n224 = Select(t=w622, s=w614, f=w623) -> (s? t:f=w621:u64)
                        n225 = Greater?(x="Number of scans", y=w621) -> (0:w607:bool)
                        n226 = Multiply(x="Scan freq.  increment", y=w617) -> (x*y=w602:i64)
                        n227 = Select(t=TRUE, s="Cont. Scan", f=w607) -> (s? t:f=w604:bool)
                        n228 = Select(t=w621, s=w604, f=w610) -> (s? t:f=w624:u64)
                        n229 = feedback-in #15(w624) -> ()
                        n230 = local read "BD 1 Frequency 1"() -> (w601:u64)
                        n231 = Increment(x=w621) -> (x+1=→"Scan I":u64)
                        n232 = Add(x=w602, y=w601) -> (x+y=w600:u64)
                        "Actual Scan freq" <- w600
                      }
                      frame True {
                        n233 = local read "Actual Scan freq"() -> (w638:u64)
                        n234 = local read "Scan steps"() -> (w639:u64)
                      }
                    }
                    "Scanning" <- w583
                    n235 = case shown="True" w575 {
                      tunnel: w578 -> [_ w599]
                      frame False {
                      }
                      frame True {
                        n236 = Add(x=w599, y=i16 2) -> (x+y=w597:u64)
                        n237 = local write "Raster to target force"(FALSE) -> ()
                        n238 = local write "Scan steps"(w597) -> ()
                      }
                    }
                  }
                }
                n239 = feedback #16(fxp<+/-,24,9> 0.0 ("AI1 X Set 2")) -> (w445:fxp<+/-,24,9>)
                n240 = Select(t=w434, s=w419, f=w445) -> (s? t:f=w446:fxp<+/-,24,9>)
                "Trap Pos FB Int Signal" <- w446
                n241 = feedback-in #16(w446) -> ()
                n242 = feedback #17(fxp<+/-,16,1> 0.0 ("Trap Pos FB Int-Norm Signal")) -> (w431:fxp<+/-,16,1>)
                n243 = Select(t=w400, s=w419, f=w431) -> (s? t:f=w430:fxp<+/-,16,1>)
                "Trap Pos FB Int-Norm Signal" <- w430
                n244 = feedback-in #17(w430) -> ()
                n245 = case "For position feedback" shown="True" "Force feedback" {
                  tunnel: [i64 0 w491] -> w425
                  tunnel: w400 -> [_ w488]
                  tunnel: w419 -> [_ w487]
                  frame False {
                  }
                  frame True {
                    n246 = feedback #18(i64 0) -> (w490:i64)
                    n247 = case shown="True" w487 {
                      tunnel: [w492 w506] -> w491
                      tunnel: w490 -> [w492 _]
                      tunnel: w488 -> [_ w500]
                      frame False {
                      }
                      frame True {
                        w510 = u32 0
                        n248 = Bundle("P2"="P2", "I2"="I2", "D2"="D2") -> (w496:T8)  [unwired: 1 in]
                        n249 = Bundle("FB2 output high"="FB2 output high", "FB2 output low"="FB2 output low") -> (w493:T9)  [unwired: 1 in]
                        n250 = xnode ("PID")("process variable"=w500, "reset?"="Trap Pos. FB Reset", "setpoint"="Trap Pos. FB SP", "PID gains"=w496, "output range"=w493) -> ("output"=w522:fxp<+/-,16,1>)
                        n251 = Negate(x=w522) -> (-x=w521:fxp<+/-,17,2>)
                        n252 = Select(t=w521, s="Trap Pos FB Negate Action", f=w522) -> (s? t:f=w518:fxp<+/-,17,2>)
                        n253 = Scale By Power Of 2(n=u32 15, x=u32 1) -> (x*2^n=w515:u32)
                        n254 = Multiply(x=w518, y=w515) -> (x*y=w514:fxp<+/-,17,17>)
                        n255 = To Quad Integer(1:w514) -> (0:w526:i64)
                        "Trap Pos FB Action" <- w526
                        n256 = Multiply(x=w526, y="Trap Pos. FB Mult Factor") -> (x*y=w524:i64)
                        n257 = Add(x=w524, y="Trap Pos. FB Offset Factor") -> (x+y=w506:i64)
                        n258 = feedback #19() -> (w507:i64)  [unwired: 1 in]
                        n259 = Add(x=w506, y=w507) -> (x+y=w504:i64)
                        n260 = feedback #20(w510) -> (w512:u32)
                        n261 = Increment(x=w512) -> (x+1=w501:u32)
                        n262 = Greater Or Equal?(x=w501, y="FB Trig Integrate") -> (x >= y?=w502:bool)
                        n263 = Select(t=i64 0, s=w502, f=w504) -> (s? t:f=w508:i64)
                        n264 = feedback-in #19(w508) -> ()
                        n265 = Select(t=w510, s=w502, f=w501) -> (s? t:f=w511:u32)
                        n266 = feedback-in #20(w511) -> ()
                        n267 = And(x=w502, y="FPGA Trap Trig") -> (x .and. y?=w509:bool)
                        n268 = case "Trap FB trigger excitation laser ON" shown="True" w509 {
                          tunnel: w504 -> [_ w530]
                          tunnel: w501 -> [_ w528]
                          frame False {
                          }
                          frame True {
                            n269 = Not(x="TTrig Negate Pos") -> (.not. x?=w537:bool)
                            n270 = Boolean To (0,1)(Boolean="TTrig Negate Pos") -> (0, 1=w535:i16)
                            n271 = Boolean To (0,1)(Boolean=w537) -> (0, 1=w536:i16)
                            n272 = Negate(x=w535) -> (-x=w534:i16)
                            n273 = Add(x=w534, y=w536) -> (x+y=w533:i16)
                            n274 = Multiply(x=w533, y=w530) -> (x*y=w532:i64)
                            "TTrig Sig" <- w532
                            n275 = Multiply(x="FPGA TTrig Thresh", y=w528) -> (x*y=w529:i64)
                            "TTrig Fin Thresh" <- w529
                            n276 = Greater Or Equal?(x=w532, y=w529) -> (x >= y?=w531:bool)
                            n277 = case shown="True" w531 {
                              frame False {
                              }
                              frame True {
                                w540 = TRUE ("Green FB On/Off")
                                w542 = u8 2 ("Operating Mode")
                                n278 = local write "Operating Mode 2"(w542) -> ()
                                n279 = local write "Operating Mode"(w542) -> ()
                                n280 = local write "Green FB On/Off"(w540) -> ()
                                n281 = local write "FPGA Trap Trig"(FALSE ("FPGA Trap Trig")) -> ()
                                "TTrig?" <- w540
                              }
                            }
                          }
                        }
                      }
                    }
                    n282 = feedback-in #18(w491) -> ()
                  }
                }
                n283 = And(x="Force feedback", y="Dynamic Force FB (Ronen)") -> (x .and. y?=w410:bool)
                n284 = case shown="False" w410 {
                  tunnel: w425 -> [w463 w467]
                  tunnel: [w462 w466] -> w404
                  tunnel: w407 -> [_ w465]
                  tunnel: w419 -> [_ w464]
                  frame False {
                    # "(BD1 Frequency 1)"
                    n285 = Add(x="BD 1 Frequency 1", y=w463) -> (x+y=w462:u64)
                  }
                  frame True {
                    n286 = case shown="False" w464 {
                      tunnel: w467 -> [_ w471]
                      tunnel: [w468 w470] -> w466
                      tunnel: w465 -> [w468 w469]
                      frame False {
                      }
                      frame True {
                        n287 = Add(x=w469, y=w471) -> (x+y=w470:u64)
                      }
                    }
                  }
                }
                n288 = case shown="True" w405 {
                  tunnel: w404 -> [w458 _]
                  tunnel: [w458 w459] -> w403
                  tunnel: w402 -> [_ w459]
                  frame False {
                  }
                  frame True {
                    n289 = local write "BD 1 Frequency 1"(w459) -> ()
                    n290 = local write "Abort scan"(FALSE) -> ()
                  }
                }
                n291 = Select(t=w449, s="Scan BD", f=w450) -> (s? t:f=w448:u64)
                n292 = Select(t=w450, s="Scan BD", f=w449) -> (s? t:f=w451:u64)
                n293 = Add(x=w448, y="BD 2 Frequency 1") -> (x+y=w453:u64)
                n294 = Compound Arithmetic op=ADD(i64 0 ("f"), w403, w451) -> (w418:u64)
                n295 = In Range and Coerce(upper limit="FB Max Frequency", x=w418, lower limit="FB Min frequency") -> (coerced(x)=w409:u64)  [unwired: 1 out]
                "BD1 Frequency Out 1" <- w409
              }
              frame 2 {
                # "Trap 2"
                n296 = case shown="False" "FB On/Off Set 2" {
                  tunnel: ["BD 1 Amplitude 2" w701] -> w680
                  tunnel: w684 -> [_ w699]
                  tunnel: w691 -> [_ w704]
                  tunnel: w690 -> [_ w703]
                  tunnel: w687 -> [_ w702]
                  tunnel: w686 -> [_ w700]
                  tunnel: w683 -> [_ w698]
                  tunnel: w682 -> [_ w697]
                  frame False {
                  }
                  frame True {
                    n297 = local read "AI2 Y Sum Set 2"() -> (w706:i16)
                    n298 = case shown="False" w700 {
                      tunnel: "FB Setpoint Set 2" -> [w712 w728]
                      tunnel: w706 -> [w713 w727]
                      tunnel: "FB Reset Set 2" -> [w714 w726]
                      tunnel: w704 -> [w710 w724]
                      tunnel: w703 -> [w711 w723]
                      tunnel: w702 -> [_ w722]
                      tunnel: [w708 w721] -> w701
                      tunnel: w699 -> [_ w720]
                      tunnel: w698 -> [_ w719]
                      tunnel: w697 -> [_ w716]
                      frame False {
                        n299 = call "Slower PID.vi"("process variable"=w713, "reset?"=w714, "setpoint"=w712, "PID gains (x 2^8)"=w710, "output range"=w711) -> ("output"=w709:i16)  [unwired: 10 out]
                        n300 = To Unsigned Word Integer(number=w709) -> (unsigned 16bit integer=w708:u16)
                      }
                      frame True {
                        n301 = call "Slower PID.vi"("process variable"=w727, "reset?"=w726, "setpoint"=w728, "PID gains (x 2^8)"=w724, "output range"=w723) -> ("output"=w725:i16)  [unwired: 10 out]
                        n302 = To Unsigned Word Integer(number=w725) -> (unsigned 16bit integer=w718:u16)
                        n303 = Scale By Power Of 2(n=w719, x=w718) -> (x*2^n=w717:u16)
                        n304 = Add(x=w717, y=w716) -> (x+y=w715:u16)
                        n305 = case shown="False" w722 {
                          tunnel: w720 -> [w730 w734]
                          tunnel: w715 -> [w729 w733]
                          tunnel: [w731 w732] -> w721
                          frame False {
                            n306 = Add(x=w730, y=w729) -> (x+y=w731:u16)
                          }
                          frame True {
                            n307 = Subtract(x=w734, y=w733) -> (x-y=w732:u16)
                          }
                        }
                      }
                    }
                  }
                }
                "BD1 measured amplitude 2" <- w680
                n308 = Add(x="BD 1 Frequency 2", y=i64 0 ("f")) -> (x+y=w689:u64)
                "BD1 Frequency Out 2" <- w689
              }
              frame 3 {
                # "Fluorescence period"
              }
            }
            n309 = feedback-in #21(w313) -> ()
            n310 = feedback #21(w313) -> (w312:u16)
            n311 = Select(t=w315, s="Interlace ON/OFF", f="Interlace Off Parameters") -> (s? t:f=w352:u8)
            n312 = Subtract(x=w313, y=w312) -> (x-y=w311:u16)
            n313 = Subtract "The error"(x=w311, y=w310) -> (x-y=w288:u16)
            n314 = case shown="1, Default" w352 {
              tunnel: ["DIO count 1 (ticks)" "DIO count 2 (ticks)" "DIO count 3 (ticks)"] -> w309
              frame 1, Default {
              }
              frame 2 {
              }
              frame 3 {
              }
            }
            n315 = Number To Boolean Array(number=w288) -> (Boolean array=w289:bool[])
            n316 = Or Array Elements(Boolean array=w289) -> (logical OR=w287:bool)
            n317 = Boolean To (0,1)(Boolean=w287) -> (0, 1=w294:i16)
            n318 = To Unsigned Byte Integer(number=w294) -> (unsigned 8bit integer=w291:u8)
            n319 = feedback #22(u8 0) -> (w292:u8)
            n320 = Add(x=w291, y=w292) -> (x+y=w290:u8)
            "DIO Late Counter" <- w290
            n321 = feedback-in #22(w290) -> ()
            n322 = Subtract(x=w309, y=w288) -> (x-y=w308:u16)
            n323 = Split Number(x=w349) -> (hi(x)=w348:u32, lo(x)=w347:u32)
            n324 = Split Number(x=w338) -> (hi(x)=w343:u32, lo(x)=w342:u32)
            n325 = Boolean To (0,1)(Boolean="+ phase (DIO)") -> (0, 1=w305:i16)
            n326 = Split Number(x=w348) -> (lo(x)=w346:u16)  [unwired: 1 out]
            n327 = Split Number(x=w347) -> (hi(x)=w345:u16, lo(x)=w344:u16)
            n328 = Split Number(x=w343) -> (lo(x)=w341:u16)  [unwired: 1 out]
            n329 = Split Number(x=w342) -> (hi(x)=w340:u16, lo(x)=w339:u16)
            n330 = Split Number(x=w298) -> (hi(x)=w300:u8, lo(x)=w299:u8)
            n331 = Split Number(x=w295) -> (hi(x)=w297:u8, lo(x)=w296:u8)
            n332 = Split Number(x=w346) -> (hi(x)=w337:u8, lo(x)=w336:u8)
            n333 = Split Number(x=w345) -> (hi(x)=w335:u8, lo(x)=w334:u8)
            n334 = Split Number(x=w341) -> (hi(x)=w330:u8, lo(x)=w329:u8)
            n335 = Split Number(x=w344) -> (hi(x)=w333:u8, lo(x)=w332:u8)
            n336 = Split Number(x=w340) -> (hi(x)=w328:u8, lo(x)=w327:u8)
            n337 = Split Number(x=w339) -> (hi(x)=w326:u8, lo(x)=w325:u8)
            n338 = Multiply(x=w305, y="Phase count adjustment (DIO)") -> (x*y=w301:i16)
            n339 = feedback #23(i16 0) -> (w303:i16)
            n340 = Subtract(x=w303, y=w301) -> (x-y=w302:i16)
            "DIO Relative phase" <- w302
            n341 = feedback-in #23(w302) -> ()
            n342 = Add(x=w308, y=w301) -> (x+y=w307:u16)
            n343 = Build Array "BD 1 A Stack"(w300, w299) -> (w322:u8[])
            n344 = Build Array "BD 2 A Stack"(w297, w296) -> (w321:u8[])
            n345 = Build Array "BD 1 nu Stack"(w337, w336, w335, w334, w333, w332) -> (w331:u8[])
            n346 = Build Array "BD 2 nu Stack"(w330, w329, w328, w327, w326, w325) -> (w324:u8[])
            n347 = case shown="2" w279 {
              tunnel: [w392 w395] -> w320
              tunnel: [u8 10 u8 4] -> w323
              tunnel: "Swap F1 and F2" -> [w393 w395]
              frame 2 {
                # "F2"
                n348 = Not(x=w393) -> (.not. x?=w392:bool)
              }
              frame 1, Default {
                # "low chooses F1"
                # "F1"
              }
            }
            n349 = case "If FPGA is controlling (toggling) RF synth" shown="True" w319 {
              tunnel: w331 -> [_ w368]
              tunnel: w324 -> [_ w367]
              tunnel: w323 -> [_ w366]
              tunnel: w322 -> [_ w365]
              tunnel: w321 -> [_ w364]
              frame False {
              }
              frame True {
                # "Write next amp.\n(wait until beginning of next loop iteration to update)"
                n350 = flat-sequence "Update the next F1 and F2 frequency value (the actual frequency won't change until FSK is switched).\nThen load the next amplitude value into buffer, but don't update it until the next cycle." {
                  tunnel: w367 -> [w370]
                  tunnel: w368 -> [w371]
                  tunnel: [w371] -> w363
                  tunnel: [w370] -> w362
                  tunnel: w366 -> [w372]
                  tunnel: w363 -> [w374]
                  tunnel: w362 -> [w373]
                  tunnel: w365 -> [w385]
                  tunnel: w364 -> [w384]
                  frame #0 {
                    # "To possibly send\nthese writes to very\nend of loop (for x and\ny phase adjust)"
                    n351 = call "Wait8"("Count(Ticks)"="Next trap write delay (ticks)") -> ()  [unwired: 1 out]
                  }
                  frame #1 {
                    n352 = for {
                      tunnel: w374 -> [w380] mode=indexing
                      tunnel: w373 -> [w379] mode=indexing
                      tunnel: w372 -> [w377]
                      i -> [w378]
                      # "Write next freq."
                      n353 = To Unsigned Byte Integer(number=w378) -> (unsigned 8bit integer=w375:u8)
                      n354 = Add(x=w377, y=w375) -> (x+y=w376:u8)
                      n355 = call "write to RF synth bd.vi"("Address Byte"=w376, "BD 2 Byte"=w379, "BD 1 Byte"=w380) -> ()
                    }
                  }
                  frame #2 {
                    w381 = TRUE ("Connector1/DIO15")
                    # "send udclk high\n(BD 1 and 2)"
                    n356 = xnode "FPGA I/O Node"("Connector1/DIO30"=w381, "Connector1/DIO29"=w381) -> ()  [unwired: 2 in, 2 out]
                  }
                  frame #3 {
                    w382 = FALSE ("Connector1/DIO15")
                    n357 = xnode "FPGA I/O Node"("Connector1/DIO30"=w382, "Connector1/DIO29"=w382) -> ()  [unwired: 2 in, 2 out]
                  }
                  frame #4 {
                    n358 = for {
                      tunnel: w385 -> [w391] mode=indexing
                      tunnel: w384 -> [w390] mode=indexing
                      tunnel: u8 33 -> [w388]
                      i -> [w389]
                      n359 = To Unsigned Byte Integer(number=w389) -> (unsigned 8bit integer=w386:u8)
                      n360 = Add(x=w388, y=w386) -> (x+y=w387:u8)
                      n361 = call "write to RF synth bd.vi"("Address Byte"=w387, "BD 2 Byte"=w390, "BD 1 Byte"=w391) -> ()
                    }
                  }
                }
              }
            }
          }
        }
      }
    }
  }
  n362 = while "APD 1 Counter" {
    tunnel: w4 -> [_]
    stop <- FALSE stop-if-true
    n363 = flat-sequence {
      frame #0 {
        n364 = xnode "FPGA I/O Method Node"("FPGA I/O In"=refnum<k21> "Connector0/DIO0" ("APD 1 DO"), "Timeout"=-1) -> ()  [unwired: 2 out]
      }
      frame #1 {
        n365 = local read "APD1 int gate"() -> (w745:bool)
        n366 = case shown="True" w745 {
          frame False {
          }
          frame True {
            n367 = local read "APD1 out state"() -> (w746:bool)
            n368 = case shown="True" w746 {
              frame False {
                n369 = local read "APD 1 Counts 0"() -> (w748:u32)
                n370 = Increment(x=w748) -> (x+1=→"APD 1 Counts 0":u32)
              }
              frame True {
                n371 = local read "APD 1 Counts 1"() -> (w750:u32)
                n372 = Increment(x=w750) -> (x+1=→"APD 1 Counts 1":u32)
              }
            }
          }
        }
      }
    }
  }
  n373 = disable-structure shown="Disabled" {
    disable-tunnel: u16 0 -> [w752 _]
    disable-tunnel: w4 -> [w751 _]
    frame Disabled {
      n374 = while "Green and red fluorescent laser interlacing (Current AO to IA 532 nm AOM ME amp)." {
        shift-right: [w761] -> _
        shift-left: w751 -> [w764]
        shift-right: [w758] -> _
        shift-left: w752 -> [w756]
        shift-right: [w755] -> _
        shift-left: w752 -> [w754]
        stop <- FALSE stop-if-true
        n375 = flat-sequence {
          tunnel: w764 -> [w768]
          tunnel: [w769] -> w763
          tunnel: [w768] -> w762
          tunnel: [w767] -> w757
          tunnel: w756 -> [w767]
          tunnel: w754 -> [w766]
          tunnel: [w766] -> w753
          tunnel: [w773] -> w760
          tunnel: w763 -> [w773]
          tunnel: [w772] -> w759
          tunnel: w762 -> [w772]
          tunnel: w757 -> [w771]
          tunnel: w753 -> [w770]
          tunnel: [w794] -> w761
          tunnel: [w810] -> w758
          tunnel: w760 -> [w821]
          tunnel: w759 -> [w818]
          tunnel: [w778] -> w755
          frame #0 {
            n376 = call "Loop Timer10"("Count(Ticks)"=w768) -> ("Tick Count(Ticks)"=w769:u16)
          }
          frame #1 {
            n377 = xnode "FPGA I/O Node"("Chassis2/Mod1/AO0"=w771, "Chassis2/Mod1/AO1"=w770) -> ()  [unwired: 2 in, 2 out]
          }
          frame #2 {
            # "Design note:\n\nThese two laser controls are in the same loop\nbecause the expansion current AI cannot separately\ntime the outputs fast enough for us.  Apparently\nit is because of communication time between the\nexpansion card and the fpga.\n\nSo the two analog control signals have the same timing\nand profile, but independent amplitudes to independently\ncontrol the intensity and feedback for each laser."
            n378 = feedback #24(TRUE) -> (w774:bool)
            n379 = Not(x=w774) -> (.not. x?=w775:bool)
            n380 = feedback-in #24(w775) -> ()
            n381 = Subtract(x="Green interlace OFF count 2", y="Green int current ON count adj") -> (x-y=w803:u16)
            n382 = feedback-in #25(w821) -> ()
            n383 = feedback #25(w821) -> (w820:u16)
            n384 = Add(x="Green int current ON count adj", y="Green interlace ON count 2") -> (x+y=w804:u16)
            n385 = Subtract(x=w821, y=w820) -> (x-y=w819:u16)
            n386 = Select(t=w804, s=w775, f=w803) -> (s? t:f=w815:u16)
            n387 = Subtract(x=w819, y=w818) -> (x-y=w787:u16)
            n388 = case shown="2" "RI Operating Mode 2" {
              tunnel: [TRUE FALSE w827] -> w776
              tunnel: w774 -> [_ _ w824]
              frame 0, Default {
              }
              frame 1 {
              }
              frame 2 {
                n389 = Not(x=w824) -> (.not. x?=w826:bool)
                n390 = Select(t=w826, s="Invert RI 2", f=w824) -> (s? t:f=w827:bool)
              }
            }
            n391 = Subtract(x=w815, y=w787) -> (x-y=w798:u16)
            n392 = case shown="0, Default" "Operating Mode 2" {
              tunnel: [TRUE FALSE w861] -> w779
              tunnel: w774 -> [_ _ w858]
              frame 0, Default {
              }
              frame 1 {
              }
              frame 2 {
                n393 = Not(x=w858) -> (.not. x?=w860:bool)
                n394 = Select(t=w860, s="Invert GI 2", f=w858) -> (s? t:f=w861:bool)
              }
            }
            n395 = Number To Boolean Array(number=w787) -> (Boolean array=w788:bool[])
            n396 = Boolean To (0,1)(Boolean="+ phase (GI) 2") -> (0, 1=w800:i16)
            n397 = Or Array Elements(Boolean array=w788) -> (logical OR=w786:bool)
            n398 = Boolean To (0,1)(Boolean=w786) -> (0, 1=w793:i16)
            n399 = Multiply(x=w800, y="Phase count adjustment (GI) 2") -> (x*y=w796:i16)
            n400 = To Unsigned Byte Integer(number=w793) -> (unsigned 8bit integer=w789:u8)
            n401 = Add(x=w798, y=w796) -> (x+y=w794:u16)
            n402 = feedback #26(u8 0) -> (w791:u8)
            n403 = Add(x=w789, y=w791) -> (x+y=w790:u8)
            "GI Late Counter 2" <- w790
            n404 = feedback-in #26(w790) -> ()
            n405 = feedback #27(i16 0) -> (w797:i16)
            n406 = Subtract(x=w797, y=w796) -> (x-y=w795:i16)
            "GI Relative phase 2" <- w795
            n407 = feedback-in #27(w795) -> ()
            n408 = And(x=w779, y="Green FB On/Off") -> (x .and. y?=w805:bool)
            n409 = And(x=w776, y="Red FB On/Off") -> (x .and. y?=w785:bool)
            n410 = case shown="False" w805 {
              tunnel: "Current Out" -> [w842 _]
              tunnel: [w842 w851] -> w809
              frame False {
              }
              frame True {
                n411 = local read "Green FB Sum"() -> (w847:i16)
                n412 = Bundle("P3"="P3", "I3"="I3", "D3"="D3") -> (w843:cluster{"P3":i16, "I3":i16, "D3":i16})  [unwired: 1 in]
                n413 = call "Slower PID.vi"("process variable"=w847, "reset?"="Green FB Reset", "setpoint"="Green FB Setpoint", "PID gains (x 2^8)"=w843, "output range"=cluster{"output high":i16, "output low":i16} {"output high"=32767, "output low"=-32768} ("Green FB output range")) -> ("output"=w854:i16)  [unwired: 10 out]
                n414 = To Long Integer(number=w854) -> (32bit integer=w848:i32)
                n415 = Add(x=w848, y=32768) -> (x+y=w850:i32)
                n416 = To Unsigned Word Integer(number=w850) -> (unsigned 16bit integer=w851:u16)
              }
            }
            n417 = case shown="True" w785 {
              tunnel: "RI Current Out" -> [w828 _]
              tunnel: [w828 w837] -> w781
              frame False {
              }
              frame True {
                n418 = local read "Red FB Intensity"() -> (w833:i16)
                n419 = Bundle("P4"="P4", "I4"="I4", "D4"="D4") -> (w829:cluster{"P4":i16, "I4":i16, "D4":i16})  [unwired: 1 in]
                n420 = call "Slower PID.vi"("process variable"=w833, "reset?"="Red FB Reset", "setpoint"="Red FB Setpoint", "PID gains (x 2^8)"=w829, "output range"=cluster{"output high":i16, "output low":i16} {"output high"=32767, "output low"=-32768} ("Green FB output range")) -> ("output"=w840:i16)  [unwired: 10 out]
                n421 = To Long Integer(number=w840) -> (32bit integer=w834:i32)
                n422 = Add(x=w834, y=32768) -> (x+y=w836:i32)
                n423 = To Unsigned Word Integer(number=w836) -> (unsigned 16bit integer=w837:u16)
              }
            }
            n424 = Boolean To (0,1)(Boolean=w779) -> (0, 1=w811:i16)
            n425 = Boolean To (0,1)(Boolean=w776) -> (0, 1=w780:i16)
            n426 = To Unsigned Word Integer(number=w811) -> (unsigned 16bit integer=w808:u16)
            n427 = To Unsigned Word Integer(number=w780) -> (unsigned 16bit integer=w782:u16)
            n428 = Multiply(x=w808, y=w809) -> (x*y=w810:u16)
            n429 = Multiply(x=w782, y=w781) -> (x*y=w778:u16)
          }
        }
      }
    }
    frame Enabled {
    }
  }
  n430 = while "APD 2 Counter" {
    tunnel: w4 -> [_]
    stop <- FALSE stop-if-true
    n431 = flat-sequence {
      frame #0 {
        n432 = xnode "FPGA I/O Method Node"("FPGA I/O In"=refnum<k21> "Connector0/DIO1" ("APD 2 DO"), "Timeout"=-1) -> ()  [unwired: 2 out]
      }
      frame #1 {
        n433 = local read "APD2 int gate"() -> (w865:bool)
        n434 = case shown="True" w865 {
          frame False {
          }
          frame True {
            n435 = local read "APD2 out state"() -> (w866:bool)
            n436 = case shown="False" w866 {
              frame False {
                n437 = local read "APD 2 Counts 0"() -> (w868:u32)
                n438 = Increment(x=w868) -> (x+1=→"APD 2 Counts 0":u32)
              }
              frame True {
                n439 = local read "APD 2 Counts 1"() -> (w870:u32)
                n440 = Increment(x=w870) -> (x+1=→"APD 2 Counts 1":u32)
              }
            }
          }
        }
      }
    }
  }
  n441 = while "532 nm green fluorescent laser interlacing (DO to IA 532 nm AOM ME amp)." {
    shift-right: [w874] -> _
    shift-left: w4 -> [w879]
    shift-right: [w873] -> _
    shift-left: w5 -> [w871]
    stop <- FALSE stop-if-true
    n442 = flat-sequence {
      tunnel: w879 -> [w882]
      tunnel: [w883] -> w877
      tunnel: [w882] -> w875
      tunnel: [w881] -> w872
      tunnel: w871 -> [w881]
      tunnel: [w886] -> w878
      tunnel: w877 -> [w886]
      tunnel: [w885] -> w876
      tunnel: w875 -> [w885]
      tunnel: w872 -> [w884]
      tunnel: [w895] -> w874
      tunnel: w878 -> [w915]
      tunnel: w876 -> [w912]
      tunnel: [w904] -> w873
      frame #0 {
        n443 = call "Loop Timer4"("Count(Ticks)"=w882) -> ("Tick Count(Ticks)"=w883:u16)
      }
      frame #1 {
        n444 = xnode "FPGA I/O Node"("Connector1/DIO34"=w884, "Connector1/DIO38"=w884, "Connector1/DIO39"=w884) -> ()  [unwired: 3 in, 3 out]
      }
      frame #2 {
        n445 = feedback-in #28(w915) -> ()
        n446 = feedback #28(w915) -> (w914:u16)
        n447 = Subtract(x=w915, y=w914) -> (x-y=w913:u16)
        n448 = Subtract(x=w913, y=w912) -> (x-y=w888:u16)
        n449 = Number To Boolean Array(number=w888) -> (Boolean array=w889:bool[])
        n450 = Or Array Elements(Boolean array=w889) -> (logical OR=w887:bool)
        n451 = Boolean To (0,1)(Boolean="+ phase (GI)") -> (0, 1=w900:i16)
        n452 = Multiply(x=w900, y="Phase count adjustment (GI)") -> (x*y=w897:i16)
        n453 = Boolean To (0,1)(Boolean=w887) -> (0, 1=w894:i16)
        n454 = To Unsigned Byte Integer(number=w894) -> (unsigned 8bit integer=w891:u8)
        n455 = feedback #29(i16 0) -> (w898:i16)
        n456 = feedback #30(u8 0) -> (w892:u8)
        n457 = Add(x=w891, y=w892) -> (x+y=w890:u8)
        "GI Late Counter" <- w890
        n458 = feedback-in #30(w890) -> ()
        n459 = Subtract(x=w898, y=w897) -> (x-y=w896:i16)
        "GI Relative phase" <- w896
        n460 = feedback-in #29(w896) -> ()
        n461 = feedback #31(TRUE) -> (w907:bool)
        n462 = case shown="2" "Operating Mode" {
          tunnel: [TRUE FALSE w921] -> w904
          tunnel: w907 -> [_ _ w918]
          frame 0, Default {
          }
          frame 1 {
          }
          frame 2 {
            n463 = Not(x=w918) -> (.not. x?=w920:bool)
            n464 = Select(t=w920, s="Invert GI", f=w918) -> (s? t:f=w921:bool)
          }
        }
        n465 = Not(x=w907) -> (.not. x?=w903:bool)
        n466 = Select(t="Green interlace ON count", s=w903, f="Green interlace OFF count") -> (s? t:f=w909:u16)
        n467 = Subtract(x=w909, y=w888) -> (x-y=w901:u16)
        n468 = Add(x=w901, y=w897) -> (x+y=w895:u16)
        n469 = feedback-in #31(w903) -> ()
      }
    }
  }
  n470 = while "Excitation laser intensity feedback measurement (all lasers)" {
    shift-right: [w922] -> _
    shift-left: w4 -> [w927]
    stop <- FALSE stop-if-true
    n471 = flat-sequence {
      tunnel: w927 -> [w929]
      tunnel: [w930] -> w925
      tunnel: [w929] -> w923
      tunnel: [w936] -> w926
      tunnel: w925 -> [w936]
      tunnel: [w935] -> w924
      tunnel: w923 -> [w935]
      tunnel: [w948] -> w922
      tunnel: w926 -> [w959]
      tunnel: w924 -> [w956]
      frame #0 {
        n472 = call "Loop Timer9"("Count(Ticks)"=w929) -> ("Tick Count(Ticks)"=w930:u16)
      }
      frame #1 {
        # "Design note:\n\nAll lasers need to be measured at the same \ntime because the AI expansion module\ncannot independently time the measurements\nwithin our requirements: their is dead time.\n\nThis probably wouldn't be an issue with the built\nin AI on the fpga board itself."
        n473 = xnode "FPGA I/O Node"("Connector1/DIO35"=TRUE) -> ("Chassis2/Mod2/AI2"=→"Blue Intensity":i16, "Chassis2/Mod2/AI1"=→"Red FB Intensity":i16, "Chassis2/Mod2/AI0"=→"Green FB Sum":i16)  [unwired: 4 in, 4 out]
      }
      frame #2 {
        n474 = feedback-in #32(w959) -> ()
        n475 = feedback #32(w959) -> (w958:u16)
        n476 = Subtract(x=w959, y=w958) -> (x-y=w957:u16)
        n477 = xnode "FPGA I/O Node"("Connector1/DIO35"=FALSE) -> ()  [unwired: 1 in, 1 out]
        n478 = Subtract(x=w957, y=w956) -> (x-y=w938:u16)
        n479 = Subtract(x="Green FB Count", y=w938) -> (x-y=w952:u16)
        n480 = Number To Boolean Array(number=w938) -> (Boolean array=w939:bool[])
        n481 = Or Array Elements(Boolean array=w939) -> (logical OR=w937:bool)
        n482 = Boolean To (0,1)(Boolean="+ phase (Green FB)") -> (0, 1=w950:i16)
        n483 = Boolean To (0,1)(Boolean=w937) -> (0, 1=w944:i16)
        n484 = Multiply(x=w950, y="Phase count adjustment (Green FB)") -> (x*y=w945:i16)
        n485 = Add(x=w952, y=w945) -> (x+y=w948:u16)
        n486 = To Unsigned Byte Integer(number=w944) -> (unsigned 8bit integer=w941:u8)
        n487 = feedback #33(i16 0) -> (w947:i16)
        n488 = Subtract(x=w947, y=w945) -> (x-y=w946:i16)
        "Green FB Relative Phase" <- w946
        n489 = feedback-in #33(w946) -> ()
        n490 = feedback #34(u8 0) -> (w942:u8)
        n491 = Add(x=w941, y=w942) -> (x+y=w940:u8)
        "Green Late Counter" <- w940
        n492 = feedback-in #34(w940) -> ()
      }
    }
  }
  n493 = while "MCL stage control" {
    shift-right: [w972] -> _
    shift-left: w4 -> [w975]
    shift-right: [w965] -> _
    shift-left: w12 -> [w962]
    shift-right: [w964] -> _
    shift-left: w11 -> [w960]
    stop <- FALSE stop-if-true
    n494 = flat-sequence {
      tunnel: w975 -> [w979]
      tunnel: [w980] -> w971
      tunnel: [w979] -> w969
      tunnel: [w978] -> w963
      tunnel: w962 -> [w978]
      tunnel: [w977] -> w961
      tunnel: w960 -> [w977]
      tunnel: w971 -> [w984]
      tunnel: [w984] -> w970
      tunnel: w969 -> [w983]
      tunnel: [w983] -> w968
      tunnel: w963 -> [w982]
      tunnel: w961 -> [w981]
      tunnel: w970 -> [w992]
      tunnel: w968 -> [w991]
      tunnel: [w992] -> w974
      tunnel: [w991] -> w973
      tunnel: [w990] -> w967
      tunnel: [w989] -> w966
      tunnel: [w1064] -> w972
      tunnel: w974 -> [w1071]
      tunnel: w973 -> [w1068]
      tunnel: w967 -> [w1066]
      tunnel: w966 -> [w1065]
      tunnel: [w1066] -> w965
      tunnel: [w1065] -> w964
      frame #0 {
        n495 = call "Loop Timer5"("Count(Ticks)"=w979) -> ("Tick Count(Ticks)"=w980:u32)
      }
      frame #1 {
        n496 = xnode "FPGA I/O Node"("Connector0/AO1"=w982, "Connector0/AO2"=w981) -> ()  [unwired: 2 in, 2 out]
      }
      frame #2 {
        n497 = local read "Scanning MCL"() -> (w1004:bool)
        n498 = Or(x=w1004, y="Start scan (MCL)") -> (x .or. y?=w999:bool)
        n499 = Not(x="Abort scan (MCL)") -> (.not. x?=w997:bool)
        n500 = And(x=w997, y=w999) -> (x .and. y?=w996:bool)
        n501 = case "Raster scan" shown="True" w996 {
          tunnel: [w1005 w1048] -> w1001
          tunnel: "Start scan (MCL)" -> [_ w1033]
          tunnel: [w1005 w1009] -> w985
          frame False {
            w1005 = i16 0
            n502 = local write "Scanning MCL"(FALSE ("scanning")) -> ()
          }
          frame True {
            w1019 = i16 0
            w1018 = u64 0
            # "scan incr."
            # "freq. incr. mult."
            # "count steps"
            # "count number of cycles"
            n503 = feedback #35(w1018) -> (w1045:u64)
            n504 = Select(t=w1018, s=w1033, f=w1045) -> (s? t:f=w1047:u64)
            n505 = Increment(x=w1047) -> (x+1=w1044:u64)
            n506 = Greater?(x="Cycles per step (MCL)", y=w1044) -> (0:w1028:bool)
            n507 = Select(t=w1044, s=w1028, f=w1018) -> (s? t:f=w1043:u64)
            n508 = feedback-in #35(w1043) -> ()
            n509 = feedback #36(w1018) -> (w1042:u64)
            n510 = Select(t=w1018, s=w1033, f=w1042) -> (s? t:f=w1037:u64)
            n511 = Increment(x=w1037) -> (x+1=w1041:u64)
            n512 = Add(x="Scan steps (MCL)", y="Scan steps (MCL)") -> (x+y=w1040:u64)
            n513 = Select(t=w1037, s=w1028, f=w1041) -> (s? t:f=w1023:u64)
            n514 = Greater?(x=w1040, y=w1023) -> (0:w1022:bool)
            n515 = Select(t=w1023, s=w1022, f=w1018) -> (s? t:f=w1038:u64)
            n516 = feedback-in #36(w1038) -> ()
            n517 = Equal?(x="Scan steps (MCL)", y=w1023) -> (x = y?=w1027:bool)
            n518 = Greater?(x="Scan steps (MCL)", y=w1037) -> (0:w1036:bool)
            n519 = feedback #37(w1019) -> (w1039:i16)
            n520 = Select(t=w1019, s=w1033, f=w1039) -> (s? t:f=w1025:i16)
            n521 = Increment(x=w1025) -> (x+1=w1035:i16)
            n522 = Decrement(x=w1025) -> (x-1=w1034:i16)
            n523 = Select(t=w1035, s=w1036, f=w1034) -> (s? t:f=w1026:i16)
            n524 = Select(t=w1025, s=w1027, f=w1026) -> (s? t:f=w1024:i16)
            n525 = Select(t=w1025, s=w1028, f=w1024) -> (s? t:f=w1020:i16)
            n526 = Select(t=w1020, s=w1022, f=w1019) -> (s? t:f=w1021:i16)
            n527 = feedback-in #37(w1021) -> ()
            n528 = feedback #38(w1018) -> (w1032:u64)
            n529 = Select(t=w1018, s=w1033, f=w1032) -> (s? t:f=w1007:u64)
            n530 = Increment(x=w1007) -> (x+1=w1029:u64)
            n531 = Select(t=w1007, s=w1022, f=w1029) -> (s? t:f=w1008:u64)
            n532 = Greater?(x="Number of scans (MCL)", y=w1008) -> (0:w1015:bool)
            n533 = Multiply(x="Scan freq.  increment (MCL)", y=w1025) -> (x*y=w1048:i16)
            n534 = Select(t=TRUE, s="Cont. Scan (MCL)", f=w1015) -> (s? t:f=w1014:bool)
            "Scanning MCL" <- w1014
            n535 = Select(t=w1008, s=w1014, f=w1018) -> (s? t:f=w1030:u64)
            n536 = feedback-in #38(w1030) -> ()
            n537 = Increment(x=w1008) -> (x+1=→"Scan I (MCL)":u64)
            n538 = To Word Integer(number=w1007) -> (16bit integer=w1010:i16)
            n539 = Multiply(x=w1010, y="Scan freq.  increment (MCL)") -> (x*y=w1009:i16)
          }
        }
        n540 = Select(t=w985, s="1D or 2D Scan?", f=i16 0) -> (s? t:f=w986:i16)
        n541 = Select(t=w986, s="MCL Scan Axis", f=w1001) -> (s? t:f=w1000:i16)
        n542 = Select(t=w1001, s="MCL Scan Axis", f=w986) -> (s? t:f=w1002:i16)
        n543 = Add(x=w1000, y="AO2") -> (x+y=w989:i16)
        n544 = Add(x="AO1", y=w1002) -> (x+y=w990:i16)
      }
      frame #3 {
        n545 = feedback-in #39(w1071) -> ()
        n546 = feedback #39(w1071) -> (w1070:u32)
        n547 = Boolean To (0,1)(Boolean="+ phase (MCL)") -> (0, 1=w1062:i16)
        n548 = Subtract(x=w1071, y=w1070) -> (x-y=w1069:u32)
        n549 = Multiply(x=w1062, y="Phase count adjustment (MCL)") -> (x*y=w1058:i16)
        n550 = Subtract(x=w1069, y=w1068) -> (x-y=w1050:u32)
        n551 = Subtract(x="MCL count", y=w1050) -> (x-y=w1060:u32)
        n552 = feedback #40(i16 0) -> (w1059:i16)
        n553 = Subtract(x=w1059, y=w1058) -> (x-y=w1057:i16)
        "MCL Relative Phase" <- w1057
        n554 = feedback-in #40(w1057) -> ()
        n555 = Number To Boolean Array(number=w1050) -> (Boolean array=w1051:bool[])
        n556 = Or Array Elements(Boolean array=w1051) -> (logical OR=w1049:bool)
        n557 = Boolean To (0,1)(Boolean=w1049) -> (0, 1=w1056:i16)
        n558 = Add(x=w1060, y=w1058) -> (x+y=w1064:u32)
        n559 = To Unsigned Byte Integer(number=w1056) -> (unsigned 8bit integer=w1053:u8)
        n560 = feedback #41(u8 0) -> (w1054:u8)
        n561 = Add(x=w1053, y=w1054) -> (x+y=w1052:u8)
        "MCL Late Counter" <- w1052
        n562 = feedback-in #41(w1052) -> ()
      }
    }
  }
  n563 = while "Control APD data integration - stream to host" {
    shift-right: [w1076] -> _
    shift-left: w8 -> [w1081]
    stop <- FALSE stop-if-true
    n564 = flat-sequence {
      tunnel: w1081 -> [w1083]
      tunnel: [w1084] -> w1079
      tunnel: [w1083] -> w1077
      tunnel: [w1094] -> w1080
      tunnel: w1079 -> [w1094]
      tunnel: [w1093] -> w1078
      tunnel: w1077 -> [w1093]
      tunnel: [w1092] -> w1075
      tunnel: [w1091] -> w1074
      tunnel: [w1085] -> w1073
      tunnel: [w1136] -> w1076
      tunnel: w1080 -> [w1146]
      tunnel: w1078 -> [w1143]
      tunnel: w1075 -> [w1129]
      tunnel: w1074 -> [w1128]
      tunnel: w1073 -> [w1116]
      frame #0 {
        n565 = call "Loop Timer6"("Count(Ticks)"=w1083) -> ("Tick Count(Ticks)"=w1084:u32)
      }
      frame #1 {
        n566 = flat-sequence {
          tunnel: [w1096] -> w1090
          tunnel: w1090 -> [w1099]
          tunnel: [w1103] -> w1089
          tunnel: [w1102] -> w1088
          tunnel: [w1099] -> w1087
          tunnel: [w1098] -> w1086
          tunnel: [w1110] -> w1091
          tunnel: [w1111] -> w1092
          tunnel: w1089 -> [w1111]
          tunnel: w1088 -> [w1110]
          tunnel: w1087 -> [w1109]
          tunnel: w1086 -> [w1108]
          tunnel: [w1108] -> w1085
          frame #0 {
            # "use separate variable so each APD won't\nhave to wait to read"
            n567 = feedback #42(FALSE) -> (w1095:bool)
            "APD1 out state" <- w1095
            "APD2 out state" <- w1095
            "APD3 out state" <- w1095
            n568 = Not(x=w1095) -> (.not. x?=w1096:bool)
            n569 = feedback-in #42(w1096) -> ()
          }
          frame #1 {
            n570 = local read "APD 3 Counts 1"() -> (w1101:u32)
            n571 = local read "APD 3 Counts 0"() -> (w1100:u32)
            n572 = local read "APD 1 Counts 1"() -> (w1107:u32)
            n573 = local read "APD 1 Counts 0"() -> (w1106:u32)
            n574 = local read "APD 2 Counts 1"() -> (w1105:u32)
            n575 = local read "APD 2 Counts 0"() -> (w1104:u32)
            n576 = Select(t=w1101, s=w1099, f=w1100) -> (s? t:f=w1098:u32)
            n577 = Select(t=w1107, s=w1099, f=w1106) -> (s? t:f=w1103:u32)
            n578 = Select(t=w1105, s=w1099, f=w1104) -> (s? t:f=w1102:u32)
          }
          frame #2 {
            n579 = case shown="False" w1109 {
              frame False {
                w1112 = u32 0 ("APD 1 Counts 0")
                n580 = local write "APD 1 Counts 0"(w1112) -> ()
                n581 = local write "APD 2 Counts 0"(w1112) -> ()
                n582 = local write "APD 3 Counts 0"(w1112) -> ()
              }
              frame True {
                w1113 = u32 0 ("APD 1 Counts 1")
                n583 = local write "APD 1 Counts 1"(w1113) -> ()
                n584 = local write "APD 2 Counts 1"(w1113) -> ()
                n585 = local write "APD 3 Counts 1"(w1113) -> ()
              }
            }
          }
        }
      }
      frame #2 {
        n586 = feedback-in #43(w1146) -> ()
        n587 = feedback #43(w1146) -> (w1145:u32)
        n588 = Subtract(x=w1146, y=w1145) -> (x-y=w1144:u32)
        n589 = Subtract(x=w1144, y=w1143) -> (x-y=w1121:u32)
        n590 = case shown="True" "APD to FIFO" {
          tunnel: w1129 -> [_ w1151]
          tunnel: w1128 -> [_ w1149]
          tunnel: w1116 -> [_ w1147]
          frame False {
          }
          frame True {
            n591 = flat-sequence {
              tunnel: 0 ("Timeout") -> [w1153]
              tunnel: w1151 -> [w1154]
              tunnel: [w1153] -> w1150
              tunnel: w1150 -> [w1155]
              tunnel: w1149 -> [w1156]
              tunnel: [w1155] -> w1148
              tunnel: w1148 -> [w1158]
              tunnel: w1147 -> [w1157]
              frame #0 {
                n592 = xnode ("FIFO Write")("Element"=w1154, "Timeout"=w1153) -> ()  [unwired: 1 in, 2 out]
              }
              frame #1 {
                n593 = xnode ("FIFO Write")("Element"=w1156, "Timeout"=w1155) -> ()  [unwired: 1 in, 2 out]
              }
              frame #2 {
                n594 = xnode ("FIFO Write")("Element"=w1157, "Timeout"=w1158) -> ()  [unwired: 1 in, 2 out]
              }
            }
          }
        }
        n595 = Subtract(x="APD Acq Rate Count", y=w1121) -> (x-y=w1137:u32)
        n596 = Number To Boolean Array(number=w1121) -> (Boolean array=w1122:bool[])
        n597 = Or Array Elements(Boolean array=w1122) -> (logical OR=w1120:bool)
        n598 = Boolean To (0,1)(Boolean=w1120) -> (0, 1=w1127:i16)
        n599 = To Unsigned Byte Integer(number=w1127) -> (unsigned 8bit integer=w1124:u8)
        n600 = feedback #44(u8 0) -> (w1125:u8)
        n601 = Add(x=w1124, y=w1125) -> (x+y=w1123:u8)
        "APD Acq Late Counter" <- w1123
        n602 = feedback-in #44(w1123) -> ()
        n603 = Boolean To (0,1)(Boolean="+ phase (APD Acq)") -> (0, 1=w1133:i16)
        n604 = Multiply(x=w1133, y="Phase Count Adjustment (APD Acq)") -> (x*y=w1130:i16)
        n605 = Add(x=w1137, y=w1130) -> (x+y=w1136:u32)
        n606 = feedback #45(i16 0) -> (w1135:i16)
        n607 = Subtract(x=w1135, y=w1130) -> (x-y=w1132:i16)
        "APD Acq Relative Phase" <- w1132
        n608 = feedback-in #45(w1132) -> ()
        n609 = To Word Integer(number=w1129) -> (16bit integer=w1138:i16)
        n610 = To Word Integer(number=w1116) -> (16bit integer=w1117:i16)
        n611 = To Word Integer(number=w1128) -> (16bit integer=w1139:i16)
        n612 = Multiply(x="APD AO scale factor", y=w1139) -> (x*y=w1118:i16)
        n613 = Multiply(x="APD AO scale factor", y=w1117) -> (x*y=w1114:i16)
        n614 = Multiply(x="APD AO scale factor", y=w1138) -> (x*y=w1119:i16)
        n615 = xnode "FPGA I/O Node"("Connector0/AO6"=w1119, "Connector0/AO7"=w1118, "Connector0/AO5"=w1114) -> ()  [unwired: 3 in, 3 out]
      }
    }
  }
  n616 = while "DAQ AI set 1" {
    shift-right: [w1159] -> _
    shift-left: w4 -> [w1164]
    stop <- FALSE stop-if-true
    n617 = flat-sequence {
      tunnel: w1164 -> [w1174]
      tunnel: [w1175] -> w1162
      tunnel: [w1174] -> w1161
      tunnel: [w1185] -> w1172
      tunnel: [w1184] -> w1171
      tunnel: [w1183] -> w1170
      tunnel: [w1182] -> w1169
      tunnel: [w1181] -> w1168
      tunnel: [w1180] -> w1167
      tunnel: [w1179] -> w1166
      tunnel: [w1178] -> w1165
      tunnel: [w1177] -> w1163
      tunnel: w1162 -> [w1177]
      tunnel: w1161 -> [w1176]
      tunnel: [w1176] -> w1160
      tunnel: [w1215] -> w1159
      tunnel: w1172 -> [w1241]
      tunnel: w1171 -> [w1207]
      tunnel: w1170 -> [w1208]
      tunnel: w1169 -> [w1187]
      tunnel: w1168 -> [w1231]
      tunnel: w1167 -> [w1230]
      tunnel: w1166 -> [w1229]
      tunnel: w1165 -> [w1228]
      tunnel: w1163 -> [w1225]
      tunnel: w1160 -> [w1222]
      frame #0 {
        n618 = call "Loop Timer3"("Count(Ticks)"=w1174) -> ("Tick Count(Ticks)"=w1175:u16)
      }
      frame #1 {
        n619 = xnode "FPGA I/O Node"("Connector1/DIO31"=TRUE ("Connector1/DIO33")) -> ("Connector0/AI0"=w1185:i16, "Connector0/AI1"=w1184:i16, "Connector0/AI2"=w1183:i16, "Connector0/AI3"=w1182:i16, "Connector0/AI4"=w1181:i16, "Connector0/AI5"=w1180:i16, "Connector0/AI6"=w1179:i16, "Connector0/AI7"=w1178:i16)  [unwired: 9 in, 9 out]
      }
      frame #2 {
        w1211 = FALSE ("AI to FIFO")
        # "Adjust phase after data acquired if button pressed"
        n620 = feedback #46(i16 1) -> (w1234:i16)
        n621 = Increment(x=w1234) -> (x+1=w1240:i16)
        n622 = Scale By Power Of 2(n="AI1 X Scale", x=w1207) -> (x*2^n=w1205:i16)
        n623 = Greater?(x=w1240, y="N of AI1 Int Acq Sets") -> (0:w1237:bool)
        n624 = Select(t=i16 1, s=w1237, f=w1240) -> (s? t:f=w1239:i16)
        n625 = feedback-in #46(w1239) -> ()
        n626 = Divide(x=w1205, y=w1187) -> (x/y=w1204:fxp<+/-,16,1>)
        n627 = feedback #47(w1211) -> (w1209:bool)
        n628 = feedback #48(w1211) -> (w1227:bool)
        n629 = case shown="2" w1234 {
          tunnel: w1208 -> [w1264 w1271 _]
          tunnel: ["Set 1" "Set 2" "Set 3"] -> w1232
          tunnel: ["AI to FIFO" w1273 w1278] -> w1226
          tunnel: w1227 -> [_ w1273 w1278]
          tunnel: ["Trap Pos to FIFO" w1272 w1277] -> w1210
          tunnel: w1209 -> [_ w1272 w1277]
          tunnel: w1204 -> [w1263 w1270 _]
          tunnel: [w1262 w1268 FALSE] -> w1191
          tunnel: [w1261 w1269 u64 0 ("BD1 Frequency Out 2")] -> w1190
          frame 1, Default {
            n630 = local read "BD1 Frequency Out 1"() -> (w1261:u64)
            n631 = Compound Arithmetic op=AND("Trap Pos to FIFO", "Set 1", "AI to FIFO") -> (w1262:bool)
            "AI2 Y Sum Set 1" <- w1264
            "AI1 X Set 1" <- w1263
          }
          frame 2 {
            n632 = local read "BD1 Frequency Out 2"() -> (w1269:u64)
            n633 = Compound Arithmetic op=AND(w1272, "Set 2", w1273) -> (w1268:bool)
            "AI2 Y Sum Set 2" <- w1271
            "AI1 X Set 2" <- w1270
          }
          frame 3 {
          }
        }
        n634 = And(x=w1232, y=w1226) -> (x .and. y?=w1233:bool)
        n635 = case shown="True" w1233 {
          tunnel: w1241 -> [_ w1292]
          tunnel: w1207 -> [_ w1291]
          tunnel: w1208 -> [_ w1290]
          tunnel: w1187 -> [_ w1289]
          tunnel: w1231 -> [_ w1288]
          tunnel: w1230 -> [_ w1287]
          tunnel: w1229 -> [_ w1286]
          tunnel: w1228 -> [_ w1285]
          tunnel: 0 ("DMA buffer timeout") -> [_ w1294]
          frame False {
          }
          frame True {
            n636 = Build Array(w1292, w1291, w1290, w1289, w1288, w1287, w1286, w1285) -> (w1293:i16[])
            n637 = for {
              tunnel: w1293 -> [w1296] mode=indexing
              tunnel: w1294 -> [w1297]
              tunnel: [w1295] -> w1283 mode=indexing
              n638 = xnode ("FIFO Write")("Element"=w1296, "Timeout"=w1297) -> ("Timed Out?"=w1295:bool)  [unwired: 1 in, 1 out]
            }
            n639 = Or Array Elements(Boolean array=w1283) -> (logical OR=w1280:bool)
            n640 = Boolean To (0,1)(Boolean=w1280) -> (0, 1=w1282:i16)
            n641 = feedback #49(u16 0) -> (w1281:u16)
            n642 = Add(x=w1282, y=w1281) -> (x+y=w1279:u16)
            "Trap AI FIFO Timeout" <- w1279
            n643 = feedback-in #49(w1279) -> ()
          }
        }
        n644 = feedback-in #47(w1210) -> ()
        n645 = feedback-in #48(w1226) -> ()
        n646 = case shown="True" w1191 {
          tunnel: w1190 -> [_ w1247]
          tunnel: [u8 0 w1244] -> w1189
          frame False {
          }
          frame True {
            n647 = Split Number(x=w1247) -> (hi(x)=w1248:u32, lo(x)=w1249:u32)
            n648 = Split Number(x=w1248) -> (lo(x)=w1250:u16)  [unwired: 1 out]
            n649 = Split Number(x=w1249) -> (hi(x)=w1251:u16, lo(x)=w1252:u16)
            n650 = Build Array "BD 1 nu Stack"(w1250, w1251, w1252) -> (w1246:u16[])
            n651 = for {
              tunnel: w1246 -> [w1259] mode=indexing
              shift-right: [w1255] -> w1244
              shift-left: u8 0 -> [w1256]
              n652 = xnode ("FIFO Method Node")("Element"=w1259, "Timeout"="Trap FIFO Set Timeout") -> ("Timed Out?"=w1258:bool)  [unwired: 1 in, 1 out]
              n653 = Boolean To (0,1)(Boolean=w1258) -> (0, 1=w1257:i16)
              n654 = To Unsigned Byte Integer(number=w1257) -> (unsigned 8bit integer=w1254:u8)
              n655 = Add(x=w1254, y=w1256) -> (x+y=w1255:u8)
            }
          }
        }
        n656 = To Unsigned Word Integer(number=w1189) -> (unsigned 16bit integer=w1188:u16)
        n657 = feedback #50(u16 0) -> (w1202:u16)
        n658 = Add(x=w1188, y=w1202) -> (x+y=w1201:u16)
        "Trap Pos FIFO Timeout" <- w1201
        n659 = feedback-in #50(w1201) -> ()
        n660 = feedback-in #51(w1225) -> ()
        n661 = feedback #51(w1225) -> (w1224:u16)
        n662 = Subtract(x=w1225, y=w1224) -> (x-y=w1223:u16)
        n663 = xnode "FPGA I/O Node"("Connector1/DIO31"=FALSE ("Connector1/DIO34")) -> ()  [unwired: 1 in, 1 out]
        n664 = Subtract(x=w1223, y=w1222) -> (x-y=w1193:u16)
        n665 = Boolean To (0,1)(Boolean="+ phase") -> (0, 1=w1218:i16)
        n666 = Multiply(x=w1218, y="Phase count adjustment") -> (x*y=w1212:i16)
        n667 = Subtract(x="ai count", y=w1193) -> (x-y=w1216:u16)
        n668 = Number To Boolean Array(number=w1193) -> (Boolean array=w1194:bool[])
        n669 = feedback #52(i16 0) -> (w1214:i16)
        n670 = Add(x=w1216, y=w1212) -> (x+y=w1215:u16)
        n671 = Subtract(x=w1214, y=w1212) -> (x-y=w1213:i16)
        "Relative phase" <- w1213
        n672 = feedback-in #52(w1213) -> ()
        n673 = Or Array Elements(Boolean array=w1194) -> (logical OR=w1192:bool)
        n674 = Boolean To (0,1)(Boolean=w1192) -> (0, 1=w1199:i16)
        n675 = To Unsigned Byte Integer(number=w1199) -> (unsigned 8bit integer=w1196:u8)
        n676 = feedback #53(u8 0) -> (w1197:u8)
        n677 = Add(x=w1196, y=w1197) -> (x+y=w1195:u8)
        "AI Late Counter" <- w1195
        n678 = feedback-in #53(w1195) -> ()
      }
    }
  }
  n679 = node-c288(w9) -> ()
  n680 = while "APD 3 Counter" {
    tunnel: w4 -> [_]
    stop <- FALSE stop-if-true
    n681 = flat-sequence {
      frame #0 {
        n682 = xnode "FPGA I/O Method Node"("FPGA I/O In"=refnum<k21> "Connector0/DIO2" ("APD 2 DO"), "Timeout"=-1) -> ()  [unwired: 2 out]
      }
      frame #1 {
        n683 = local read "APD3 int gate"() -> (w1301:bool)
        n684 = case shown="True" w1301 {
          frame False {
          }
          frame True {
            n685 = local read "APD3 out state"() -> (w1302:bool)
            n686 = case shown="True" w1302 {
              frame False {
                n687 = local read "APD 3 Counts 0"() -> (w1304:u32)
                n688 = Increment(x=w1304) -> (x+1=→"APD 3 Counts 0":u32)
              }
              frame True {
                n689 = local read "APD 3 Counts 1"() -> (w1306:u32)
                n690 = Increment(x=w1306) -> (x+1=→"APD 3 Counts 1":u32)
              }
            }
          }
        }
      }
    }
  }
  n691 = while "APD 3 Gating" {
    shift-right: [w1310] -> _
    shift-left: w4 -> [w1315]
    shift-right: [w1309] -> _
    shift-left: w7 -> [w1307]
    stop <- FALSE stop-if-true
    n692 = flat-sequence {
      tunnel: w1315 -> [w1318]
      tunnel: [w1319] -> w1313
      tunnel: [w1318] -> w1311
      tunnel: [w1317] -> w1308
      tunnel: w1307 -> [w1317]
      tunnel: [w1322] -> w1314
      tunnel: w1313 -> [w1322]
      tunnel: [w1321] -> w1312
      tunnel: w1311 -> [w1321]
      tunnel: w1308 -> [w1320]
      tunnel: [w1343] -> w1310
      tunnel: w1314 -> [w1354]
      tunnel: w1312 -> [w1351]
      tunnel: [w1323] -> w1309
      frame #0 {
        n693 = call "Loop Timer15"("Count(Ticks)"=w1318) -> ("Tick Count(Ticks)"=w1319:u16)
      }
      frame #1 {
        # "Signal maybe then sent through \na transistor before APD"
        n694 = xnode "FPGA I/O Node"("Connector0/DIO12"=w1320, "Connector0/DIO13"=w1320, "Connector0/DIO14"=w1320, "Connector0/DIO15"=w1320) -> ()  [unwired: 4 in, 4 out]
        "APD3 int gate" <- w1320
      }
      frame #2 {
        n695 = local read "APD Gate OFF Count"() -> (w1328:u16)
        n696 = local read "APD Gate ON Count"() -> (w1329:u16)
        n697 = feedback #54(TRUE) -> (w1348:bool)
        n698 = feedback-in #55(w1354) -> ()
        n699 = feedback #55(w1354) -> (w1353:u16)
        n700 = Not(x=w1348) -> (.not. x?=w1346:bool)
        n701 = feedback-in #54(w1346) -> ()
        n702 = Subtract(x=w1354, y=w1353) -> (x-y=w1352:u16)
        n703 = Select(t=w1329, s=w1346, f=w1328) -> (s? t:f=w1350:u16)
        n704 = Subtract(x=w1352, y=w1351) -> (x-y=w1331:u16)
        n705 = Subtract(x=w1350, y=w1331) -> (x-y=w1342:u16)
        n706 = Number To Boolean Array(number=w1331) -> (Boolean array=w1332:bool[])
        n707 = Or Array Elements(Boolean array=w1332) -> (logical OR=w1330:bool)
        n708 = Boolean To (0,1)(Boolean=w1330) -> (0, 1=w1337:i16)
        n709 = Boolean To (0,1)(Boolean="+ phase (APD 3 Gate)") -> (0, 1=w1340:i16)
        n710 = To Unsigned Byte Integer(number=w1337) -> (unsigned 8bit integer=w1334:u8)
        n711 = Multiply(x=w1340, y="Phase count adjustment (APD 3 Gate)") -> (x*y=w1338:i16)
        n712 = feedback #56(u8 0) -> (w1335:u8)
        n713 = Add(x=w1334, y=w1335) -> (x+y=w1333:u8)
        "APD 3 Gate Late Counter" <- w1333
        n714 = feedback-in #56(w1333) -> ()
        n715 = Add(x=w1342, y=w1338) -> (x+y=w1343:u16)
        n716 = feedback #57(i16 0) -> (w1345:i16)
        n717 = Subtract(x=w1345, y=w1338) -> (x-y=w1344:i16)
        "APD 3 Gate Relative Phase" <- w1344
        n718 = feedback-in #57(w1344) -> ()
        n719 = local read "APD Gate Operating Mode"() -> (w1327:u8)
        n720 = case shown="2" w1327 {
          tunnel: [TRUE FALSE w1357] -> w1324
          tunnel: w1348 -> [_ _ w1357]
          frame 0, Default {
          }
          frame 1 {
          }
          frame 2 {
          }
        }
        n721 = local read "Invert APD Gate"() -> (w1326:bool)
        n722 = Not(x=w1324) -> (.not. x?=w1325:bool)
        n723 = Select(t=w1325, s=w1326, f=w1324) -> (s? t:f=w1323:bool)
      }
    }
  }
  n724 = disable-structure shown="Disabled" {
    disable-tunnel: w5 -> [w1359 _]
    disable-tunnel: w4 -> [w1358 _]
    frame Disabled {
      n725 = while "633 nm red  fluorescent laser interlacing (DO to IA 633 nm AOM ME amp)." {
        shift-right: [w1363] -> _
        shift-left: w1358 -> [w1368]
        shift-right: [w1362] -> _
        shift-left: w1359 -> [w1360]
        stop <- FALSE stop-if-true
        n726 = flat-sequence {
          tunnel: w1368 -> [w1371]
          tunnel: [w1372] -> w1366
          tunnel: [w1371] -> w1364
          tunnel: [w1370] -> w1361
          tunnel: w1360 -> [w1370]
          tunnel: [w1375] -> w1367
          tunnel: w1366 -> [w1375]
          tunnel: [w1374] -> w1365
          tunnel: w1364 -> [w1374]
          tunnel: w1361 -> [w1373]
          tunnel: [w1384] -> w1363
          tunnel: w1367 -> [w1404]
          tunnel: w1365 -> [w1401]
          tunnel: [w1393] -> w1362
          frame #0 {
            n727 = call "Loop Timer11"("Count(Ticks)"=w1371) -> ("Tick Count(Ticks)"=w1372:u16)
          }
          frame #1 {
            # "Then to PRL 440 amp"
            n728 = xnode "FPGA I/O Node"("Connector1/DIO32"=w1373) -> ()  [unwired: 1 in, 1 out]
          }
          frame #2 {
            n729 = feedback-in #58(w1404) -> ()
            n730 = feedback #58(w1404) -> (w1403:u16)
            n731 = Subtract(x=w1404, y=w1403) -> (x-y=w1402:u16)
            n732 = Subtract(x=w1402, y=w1401) -> (x-y=w1377:u16)
            n733 = Number To Boolean Array(number=w1377) -> (Boolean array=w1378:bool[])
            n734 = Or Array Elements(Boolean array=w1378) -> (logical OR=w1376:bool)
            n735 = Boolean To (0,1)(Boolean="+ phase (RI)") -> (0, 1=w1389:i16)
            n736 = Multiply(x=w1389, y="Phase count adjustment (RI)") -> (x*y=w1386:i16)
            n737 = Boolean To (0,1)(Boolean=w1376) -> (0, 1=w1383:i16)
            n738 = To Unsigned Byte Integer(number=w1383) -> (unsigned 8bit integer=w1380:u8)
            n739 = feedback #59(i16 0) -> (w1387:i16)
            n740 = feedback #60(u8 0) -> (w1381:u8)
            n741 = Add(x=w1380, y=w1381) -> (x+y=w1379:u8)
            "RI Late Counter" <- w1379
            n742 = feedback-in #60(w1379) -> ()
            n743 = Subtract(x=w1387, y=w1386) -> (x-y=w1385:i16)
            "RI Relative phase" <- w1385
            n744 = feedback-in #59(w1385) -> ()
            n745 = feedback #61(TRUE) -> (w1396:bool)
            n746 = case shown="2" "Red Laser Operating Mode" {
              tunnel: [TRUE FALSE w1410] -> w1393
              tunnel: w1396 -> [_ _ w1407]
              frame 0, Default {
              }
              frame 1 {
              }
              frame 2 {
                n747 = Not(x=w1407) -> (.not. x?=w1409:bool)
                n748 = Select(t=w1409, s="Invert RI", f=w1407) -> (s? t:f=w1410:bool)
              }
            }
            n749 = Not(x=w1396) -> (.not. x?=w1392:bool)
            n750 = Select(t="Red interlace ON count", s=w1392, f="Red interlace OFF count") -> (s? t:f=w1398:u16)
            n751 = Subtract(x=w1398, y=w1377) -> (x-y=w1390:u16)
            n752 = Add(x=w1390, y=w1386) -> (x+y=w1384:u16)
            n753 = feedback-in #61(w1392) -> ()
          }
        }
      }
    }
    frame Enabled {
    }
  }
  n754 = disable-structure shown="Disabled" {
    disable-tunnel: w4 -> [w1411 _]
    frame Disabled {
      n755 = while "Blue fluorescent laser interlacing (AO control direct to laser)." {
        shift-right: [w1418] -> _
        shift-left: w1411 -> [w1421]
        shift-right: [w1415] -> _
        shift-left: i16 0 -> [w1413]
        stop <- FALSE stop-if-true
        n756 = flat-sequence {
          tunnel: w1421 -> [w1424]
          tunnel: [w1425] -> w1420
          tunnel: [w1424] -> w1419
          tunnel: [w1423] -> w1414
          tunnel: w1413 -> [w1423]
          tunnel: [w1428] -> w1417
          tunnel: w1420 -> [w1428]
          tunnel: [w1427] -> w1416
          tunnel: w1419 -> [w1427]
          tunnel: w1414 -> [w1426]
          tunnel: [w1438] -> w1418
          tunnel: [w1454] -> w1415
          tunnel: w1417 -> [w1466]
          tunnel: w1416 -> [w1463]
          frame #0 {
            n757 = call "Loop Timer13"("Count(Ticks)"=w1424) -> ("Tick Count(Ticks)"=w1425:u16)
          }
          frame #1 {
            n758 = xnode "FPGA I/O Node"("Connector0/AO3"=w1426) -> ()  [unwired: 1 in, 1 out]
          }
          frame #2 {
            n759 = Subtract(x="Blue OFF count (AO)", y="Blue current ON count adj (AO)") -> (x-y=w1447:u16)
            n760 = feedback-in #62(w1466) -> ()
            n761 = feedback #62(w1466) -> (w1465:u16)
            n762 = Add(x="Blue current ON count adj (AO)", y="Blue ON count (AO)") -> (x+y=w1448:u16)
            n763 = Subtract(x=w1466, y=w1465) -> (x-y=w1464:u16)
            n764 = Subtract(x=w1464, y=w1463) -> (x-y=w1431:u16)
            n765 = Number To Boolean Array(number=w1431) -> (Boolean array=w1432:bool[])
            n766 = Boolean To (0,1)(Boolean="+ phase (BI AO)") -> (0, 1=w1444:i16)
            n767 = Or Array Elements(Boolean array=w1432) -> (logical OR=w1430:bool)
            n768 = Boolean To (0,1)(Boolean=w1430) -> (0, 1=w1437:i16)
            n769 = Multiply(x=w1444, y="Phase count adjustment (BI AO)") -> (x*y=w1440:i16)
            n770 = To Unsigned Byte Integer(number=w1437) -> (unsigned 8bit integer=w1433:u8)
            n771 = feedback #63(u8 0) -> (w1435:u8)
            n772 = Add(x=w1433, y=w1435) -> (x+y=w1434:u8)
            "BI Late Counter (AO)" <- w1434
            n773 = feedback-in #63(w1434) -> ()
            n774 = feedback #64(i16 0) -> (w1441:i16)
            n775 = Subtract(x=w1441, y=w1440) -> (x-y=w1439:i16)
            "BI Relative phase (AO)" <- w1439
            n776 = feedback-in #64(w1439) -> ()
            n777 = feedback #65(TRUE) -> (w1458:bool)
            n778 = case shown="2" "BI Operating Mode (AO)" {
              tunnel: [TRUE FALSE w1482] -> w1449
              tunnel: w1458 -> [_ _ w1479]
              frame 0, Default {
              }
              frame 1 {
              }
              frame 2 {
                n779 = Not(x=w1479) -> (.not. x?=w1481:bool)
                n780 = Select(t=w1481, s="Invert BI (AO)", f=w1479) -> (s? t:f=w1482:bool)
              }
            }
            n781 = And(x=w1449, y="Blue FB On/Off") -> (x .and. y?=w1450:bool)
            n782 = case shown="True" w1450 {
              tunnel: "BI Current Out" -> [w1467 _]
              tunnel: [w1467 w1469] -> w1453
              frame False {
              }
              frame True {
                n783 = local read "Blue Intensity"() -> (w1468:i16)
                n784 = Bundle("P5"="P5", "I5"="I5", "D5"="D5") -> (w1470:cluster{"P5":i16, "I5":i16, "D5":i16})  [unwired: 1 in]
                n785 = call "Slower PID.vi"("process variable"=w1468, "reset?"="Blue FB Reset", "setpoint"="Blue FB Setpoint", "PID gains (x 2^8)"=w1470, "output range"=cluster{"output high":i16, "output low":i16} {"output high"=32767, "output low"=0} ("Green FB output range")) -> ("output"=w1469:i16)  [unwired: 10 out]
              }
            }
            n786 = Not(x=w1458) -> (.not. x?=w1455:bool)
            n787 = Select(t=w1448, s=w1455, f=w1447) -> (s? t:f=w1460:u16)
            n788 = Subtract(x=w1460, y=w1431) -> (x-y=w1442:u16)
            n789 = Add(x=w1442, y=w1440) -> (x+y=w1438:u16)
            n790 = feedback-in #65(w1455) -> ()
            n791 = Boolean To (0,1)(Boolean=w1449) -> (0, 1=w1429:i16)
            n792 = Multiply(x=w1429, y=w1453) -> (x*y=w1454:i16)
          }
        }
      }
    }
    frame Enabled {
    }
  }
  n793 = disable-structure shown="Disabled" {
    disable-tunnel: w5 -> [w1484 _]
    disable-tunnel: w4 -> [w1483 _]
    frame Disabled {
      n794 = while "473 nm blue  fluorescent laser interlacing (DO to blue laser digital control input)." {
        shift-right: [w1488] -> _
        shift-left: w1483 -> [w1493]
        shift-right: [w1487] -> _
        shift-left: w1484 -> [w1485]
        stop <- FALSE stop-if-true
        n795 = flat-sequence {
          tunnel: w1493 -> [w1496]
          tunnel: [w1497] -> w1491
          tunnel: [w1496] -> w1489
          tunnel: [w1495] -> w1486
          tunnel: w1485 -> [w1495]
          tunnel: [w1500] -> w1492
          tunnel: w1491 -> [w1500]
          tunnel: [w1499] -> w1490
          tunnel: w1489 -> [w1499]
          tunnel: w1486 -> [w1498]
          tunnel: [w1509] -> w1488
          tunnel: w1492 -> [w1529]
          tunnel: w1490 -> [w1526]
          tunnel: [w1518] -> w1487
          frame #0 {
            n796 = call "Loop Timer14"("Count(Ticks)"=w1496) -> ("Tick Count(Ticks)"=w1497:u16)
          }
          frame #1 {
            n797 = xnode "FPGA I/O Node"("Connector1/DIO28"=w1498) -> ()  [unwired: 1 in, 1 out]
          }
          frame #2 {
            n798 = feedback-in #66(w1529) -> ()
            n799 = feedback #66(w1529) -> (w1528:u16)
            n800 = Subtract(x=w1529, y=w1528) -> (x-y=w1527:u16)
            n801 = Subtract(x=w1527, y=w1526) -> (x-y=w1502:u16)
            n802 = Number To Boolean Array(number=w1502) -> (Boolean array=w1503:bool[])
            n803 = Or Array Elements(Boolean array=w1503) -> (logical OR=w1501:bool)
            n804 = Boolean To (0,1)(Boolean="+ phase (BI D)") -> (0, 1=w1514:i16)
            n805 = Multiply(x=w1514, y="Phase count adjustment (BI D)") -> (x*y=w1511:i16)
            n806 = Boolean To (0,1)(Boolean=w1501) -> (0, 1=w1508:i16)
            n807 = To Unsigned Byte Integer(number=w1508) -> (unsigned 8bit integer=w1505:u8)
            n808 = feedback #67(i16 0) -> (w1512:i16)
            n809 = feedback #68(u8 0) -> (w1506:u8)
            n810 = Add(x=w1505, y=w1506) -> (x+y=w1504:u8)
            "Blue Late Counter (D)" <- w1504
            n811 = feedback-in #68(w1504) -> ()
            n812 = Subtract(x=w1512, y=w1511) -> (x-y=w1510:i16)
            "BI Relative phase (D)" <- w1510
            n813 = feedback-in #67(w1510) -> ()
            n814 = feedback #69(TRUE) -> (w1521:bool)
            n815 = case shown="2" "Blue Laser Operating Mode (D)" {
              tunnel: [TRUE FALSE w1535] -> w1518
              tunnel: w1521 -> [_ _ w1532]
              frame 0, Default {
              }
              frame 1 {
              }
              frame 2 {
                n816 = Not(x=w1532) -> (.not. x?=w1534:bool)
                n817 = Select(t=w1534, s="Invert BI (D)", f=w1532) -> (s? t:f=w1535:bool)
              }
            }
            n818 = Not(x=w1521) -> (.not. x?=w1517:bool)
            n819 = Select(t="Blue interlace ON count (D)", s=w1517, f="Blue interlace OFF count (D)") -> (s? t:f=w1523:u16)
            n820 = Subtract(x=w1523, y=w1502) -> (x-y=w1515:u16)
            n821 = Add(x=w1515, y=w1511) -> (x+y=w1509:u16)
            n822 = feedback-in #69(w1517) -> ()
          }
        }
      }
    }
    frame Enabled {
    }
  }
